vi "Condition _string_For_Month.vi"(0 "Select Line 2":string(combo)="ST 1", 1 "connection reference":T1, 2 "Shift":string(combo)="ALL", 3 "BREAKDOWN_STK_HOLD_ID":i32=1, 4 "Found Date":string[](array[string]), 5 "year":string(combo)="ST 1", 6 "month":string, 7 "error in (no error)":errorcluster) -> (12 "Duration count":string[][](array[string]), 13 "error out":errorcluster, 15 "connection reference 2":T1, 18 "BD Count":string[][](array[string]))   [LabVIEW 2017]
uses:
  <vilib>/addons/database/Connection.llb/Conn ObjectReference.ctl
  <vilib>/addons/database/NI_Database_API.lvlib
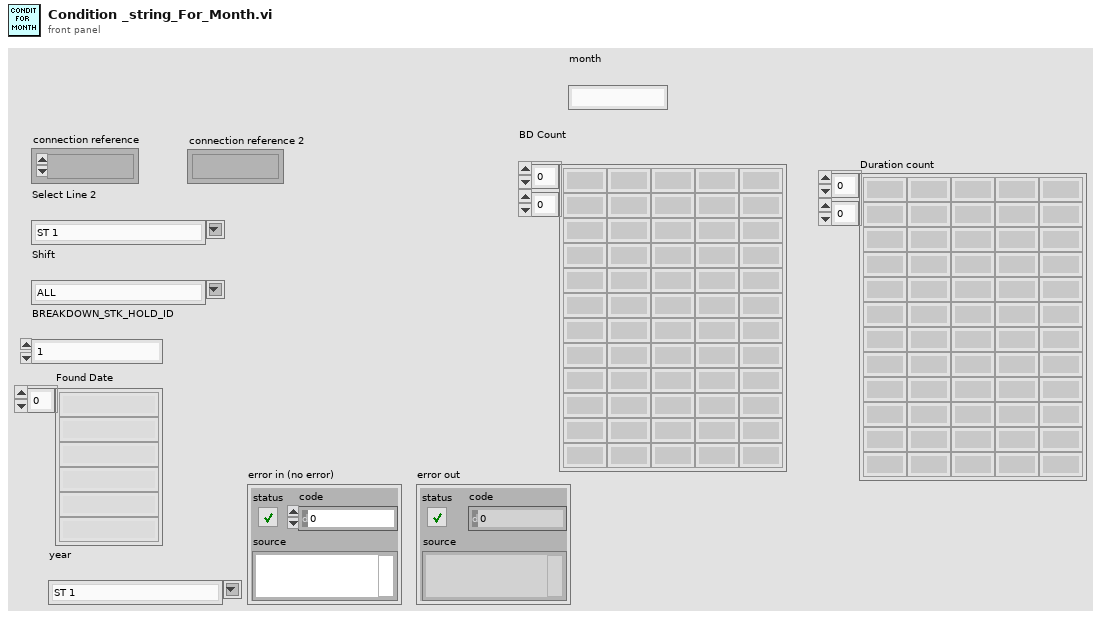
[diagram p1: front panel]
types:
  T1 = typedef "NI_Database_API.lvlib/Conn ObjectReference.ctl" = refnum<k1>
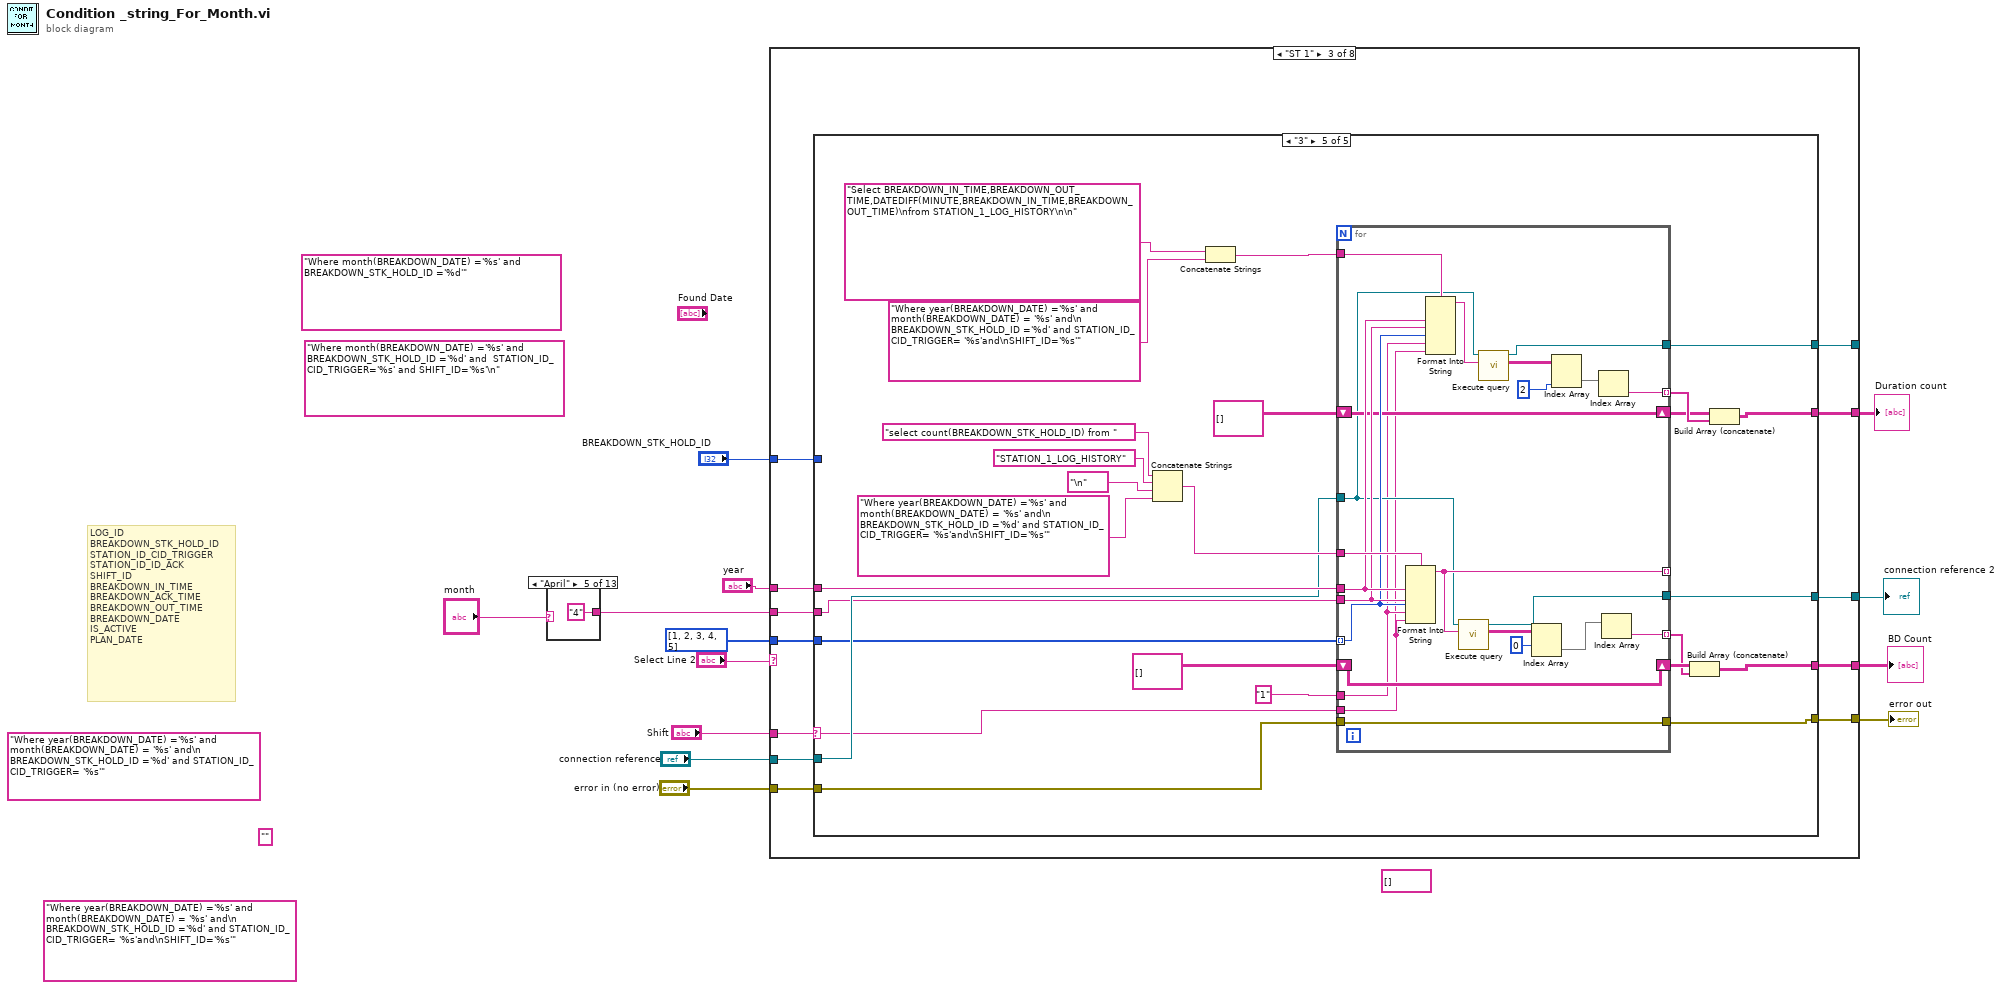
[diagram p0: block diagram]
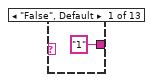
[diagram p2: hidden frame]
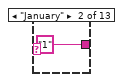
[diagram p3: hidden frame]
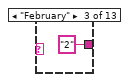
[diagram p4: hidden frame]
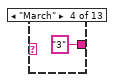
[diagram p5: hidden frame]
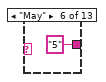
[diagram p6: hidden frame]
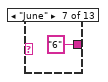
[diagram p7: hidden frame]
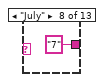
[diagram p8: hidden frame]
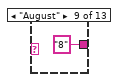
[diagram p9: hidden frame]
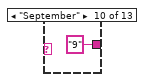
[diagram p10: hidden frame]
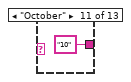
[diagram p11: hidden frame]
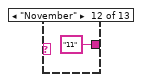
[diagram p12: hidden frame]
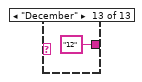
[diagram p13: hidden frame]
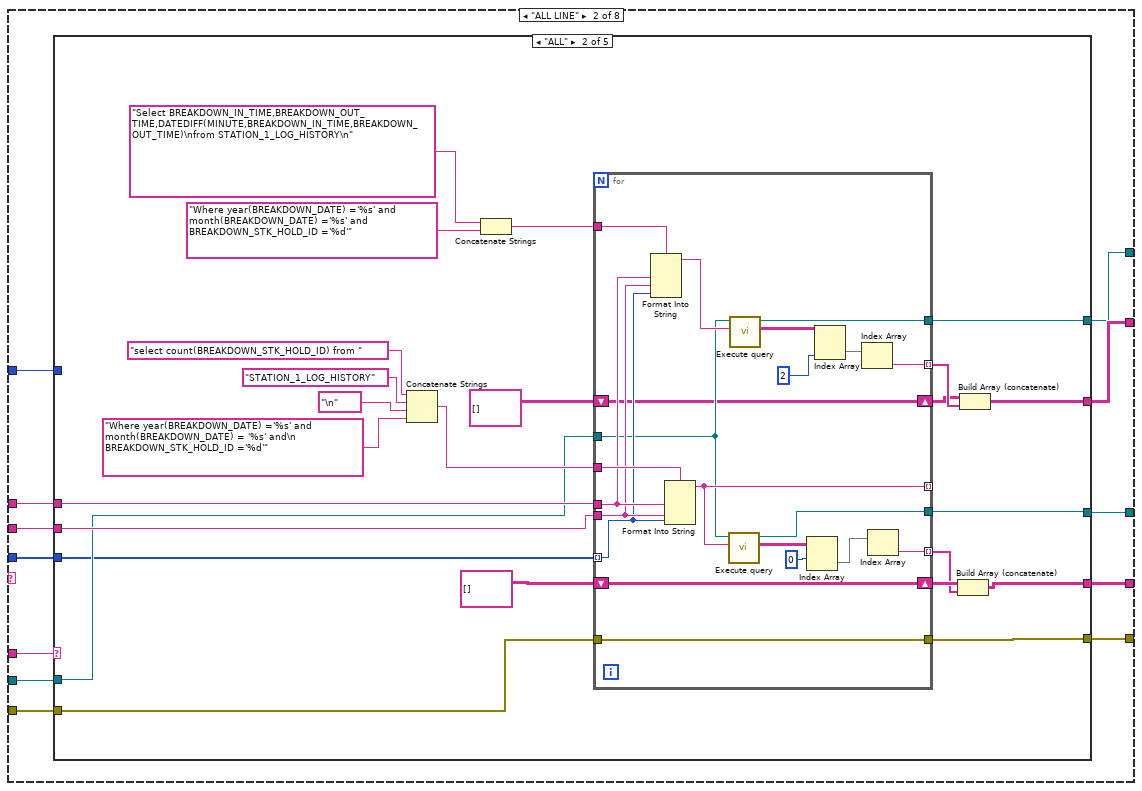
[diagram p15: hidden frame]
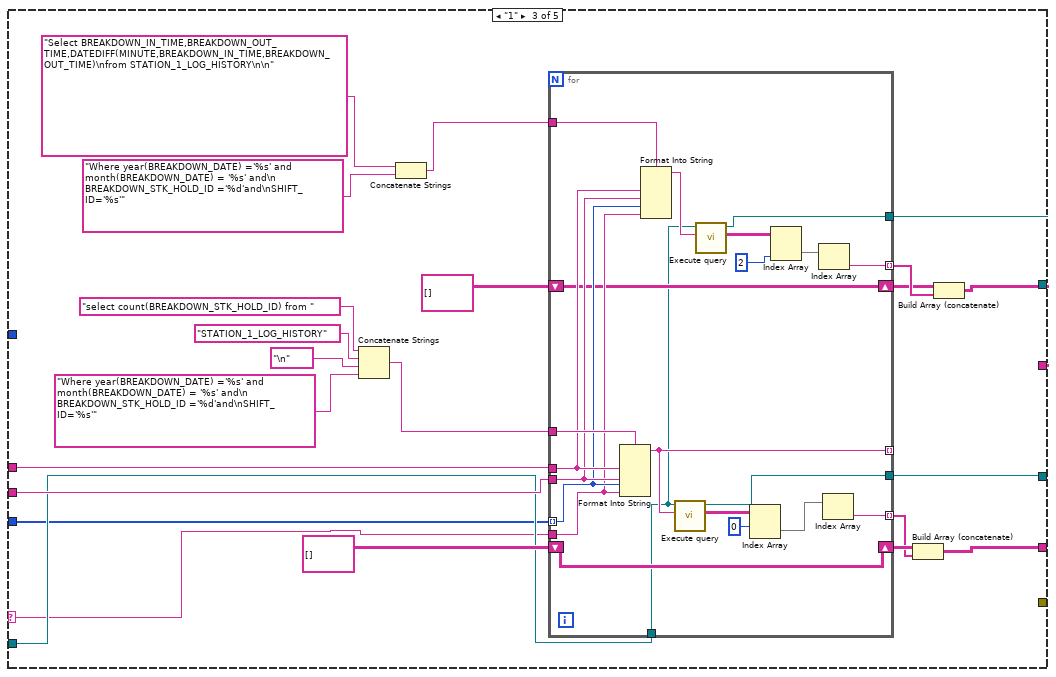
[diagram p17: hidden frame]
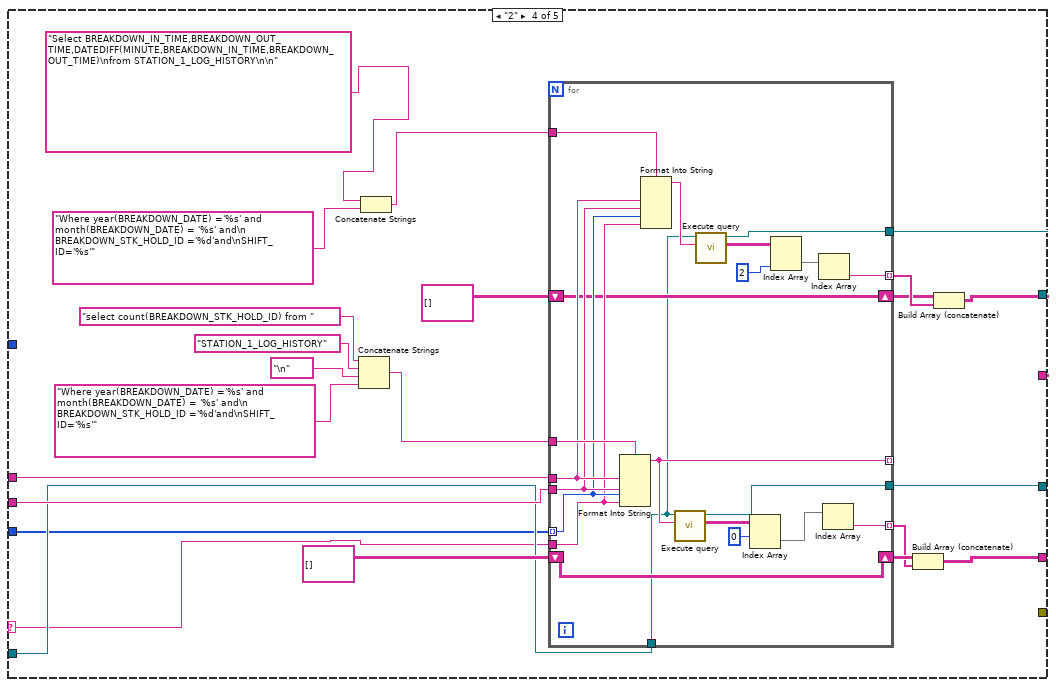
[diagram p18: hidden frame]
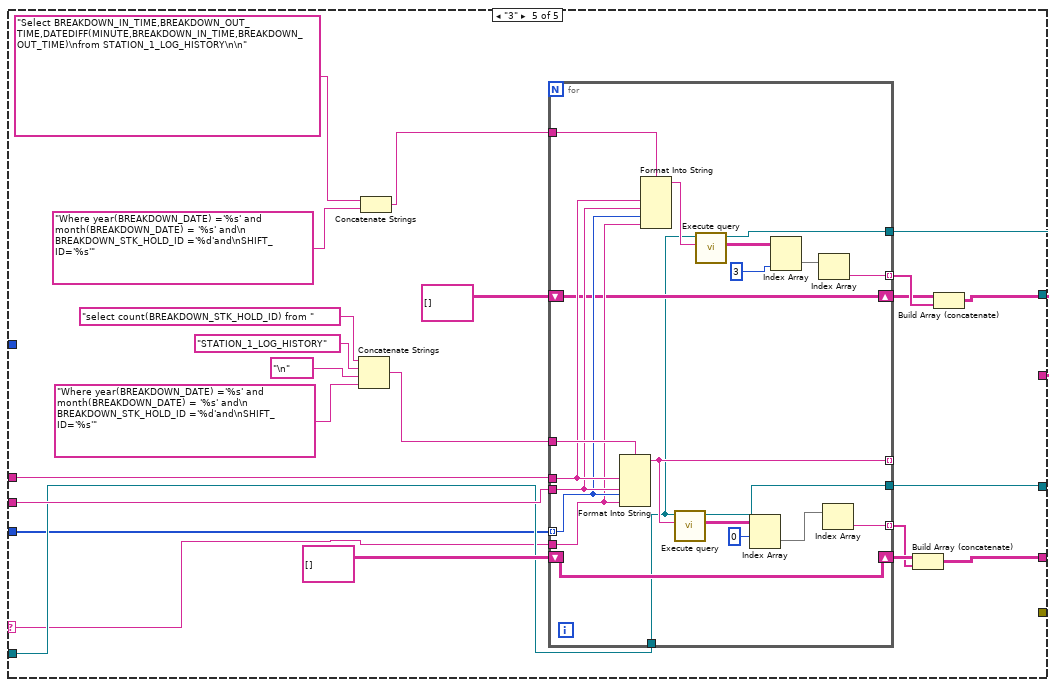
[diagram p19: hidden frame]
diagram:
  (unwired) "Where month(BREAKDOWN_DATE) ='%s' and  BREAKDOWN_STK_HOLD_ID ='%d'" ("condition")
  (unwired) "Where month(BREAKDOWN_DATE) ='%s' and  BREAKDOWN_STK_HOLD_ID ='%d' and  STATION_ID_CID_TRIGGER='%s' and SHIFT_ID='%s'\n" ("condition")
  (unwired) ""
  (unwired) "Where year(BREAKDOWN_DATE) ='%s' and month(BREAKDOWN_DATE) = '%s' and\n BREAKDOWN_STK_HOLD_ID ='%d' and STATION_ID_CID_TRIGGER= '%s'and\nSHIFT_ID='%s'" ("condition")
  (unwired) "Where year(BREAKDOWN_DATE) ='%s' and month(BREAKDOWN_DATE) = '%s' and\n BREAKDOWN_STK_HOLD_ID ='%d' and STATION_ID_CID_TRIGGER= '%s'" ("condition")
  (unwired) string[] [] ("Output Array")
  # "LOG_ID\nBREAKDOWN_STK_HOLD_ID\nSTATION_ID_CID_TRIGGER\nSTATION_ID_ID_ACK\nSHIFT_ID\nBREAKDOWN_IN_TIME\nBREAKDOWN_ACK_TIME\nBREAKDOWN_OUT_TIME\nBREAKDOWN_DATE\nIS_ACTIVE\nPLAN_DATE"
  n1 = case shown="\"April\"" "month" {
    tunnel: ["1" "1" "2" "3" "4" "5" "6" "7" "8" "9" "10" "11" "12"] -> w1
    frame "False", Default {
    }
    frame "January" {
    }
    frame "February" {
    }
    frame "March" {
    }
    frame "April" {
    }
    frame "May" {
    }
    frame "June" {
    }
    frame "July" {
    }
    frame "August" {
    }
    frame "September" {
    }
    frame "October" {
    }
    frame "November" {
    }
    frame "December" {
    }
  }
  n2 = case shown="\"ST 1\"" "Select Line 2" {
    tunnel: "Shift" -> [_ w38 w229 w437 w717 w997 w1277 w1560]
    tunnel: "BREAKDOWN_STK_HOLD_ID" -> [_ w37 w228 w436 w716 w996 w1276 w1559]
    tunnel: "year" -> [_ w36 w227 w435 w715 w995 w1275 w1558]
    tunnel: w1 -> [_ w35 w226 w434 w714 w994 w1274 w1557]
    tunnel: [_ w34 w225 w433 w713 w993 w1273 w1556] -> w9
    tunnel: "connection reference" -> [_ w33 w224 w432 w712 w992 w1272 w1555]
    tunnel: [_ w32 w223 w431 w711 w991 w1271 w1554] -> w7
    tunnel: i32[] [1, 2, 3, 4, 5] -> [_ w31 w222 w430 w710 w990 w1270 w1553]
    tunnel: [_ w30 w221 w429 w709 w989 w1269 w1552] -> w5
    tunnel: [_ w29 w220 w428 w708 w988 w1268 w1551] -> _
    tunnel: "error in (no error)" -> [_ w28 w219 w427 w707 w987 w1267 w1550]
    tunnel: [_ w27 w218 w426 w706 w986 w1266 w1549] -> w3
    frame "False", Default {
    }
    frame "ALL LINE" {
      n3 = case shown="\"ALL\"" w38 {
        selector: w38 -> [_ _ w96 w140 w184]
        tunnel: w37 -> [_ _ _ _ _]
        tunnel: w36 -> [_ w59 w103 w147 w191]
        tunnel: w35 -> [_ w56 w100 w144 w188]
        tunnel: [_ w60 w104 w148 w192] -> w34
        tunnel: w33 -> [w40 w55 w99 w143 w187]
        tunnel: [w40 w54 w98 w142 w186] -> w32
        tunnel: w31 -> [_ w53 w97 w141 w185]
        tunnel: [_ w49 w93 w136 w180] -> w30
        tunnel: [_ w48 w92 w135 w179] -> w29
        tunnel: w28 -> [w39 w46 _ _ _]
        tunnel: [w39 w45 _ _ _] -> w27
        frame "False", Default {
        }
        frame "ALL" {
          n4 = Concatenate Strings("select count(BREAKDOWN_STK_HOLD_ID) from " ("string"), "STATION_1_LOG_HISTORY" ("table"), "\n" ("string"), "Where year(BREAKDOWN_DATE) ='%s' and month(BREAKDOWN_DATE) = '%s' and\n BREAKDOWN_STK_HOLD_ID ='%d'" ("condition")) -> (w58:string)
          n5 = Concatenate Strings("Select BREAKDOWN_IN_TIME,BREAKDOWN_OUT_TIME,DATEDIFF(MINUTE,BREAKDOWN_IN_TIME,BREAKDOWN_OUT_TIME)\nfrom STATION_1_LOG_HISTORY\n" ("string"), "Where year(BREAKDOWN_DATE) ='%s' and month(BREAKDOWN_DATE) ='%s' and BREAKDOWN_STK_HOLD_ID ='%d'" ("condition")) -> (w51:string)
          n6 = for {
            tunnel: w58 -> [w85]
            tunnel: w59 -> [w75]
            tunnel: w56 -> [w74]
            tunnel: [w84] -> _ mode=indexing
            tunnel: w55 -> [w72]
            tunnel: [w82] -> w54
            tunnel: w53 -> [w73] mode=indexing
            shift-right: [w83] -> w44
            shift-left: string[][] [] ("Output Array") -> [w83]
            tunnel: [w78] -> w43 mode=indexing
            tunnel: w51 -> [w76]
            tunnel: [w69] -> w48
            tunnel: [w68] -> w42 mode=indexing
            shift-right: [w67] -> w41
            shift-left: string[][] [] ("Output Array") -> [w67]
            tunnel: [w65] -> w45
            tunnel: w46 -> [w65]
            n7 = Format Into String(format string=w76, w75, w74, w73) -> (resulting string=w77:string)  [unwired: 2 in, 1 out]
            n8 = Format Into String(format string=w85, w75, w74, w73) -> (resulting string=w84:string)  [unwired: 2 in, 1 out]
            n9 = call "Execute query.vi"("String"=w84, "connection reference"=w72) -> ("Table"=w81:string[][], "connection reference 2"=w82:T1)  [unwired: 6 in, 2 out]
            n10 = call "Execute query.vi"("String"=w77, "connection reference"=w72) -> ("Table"=w71:string[][], "connection reference 2"=w69:T1)  [unwired: 6 in, 2 out]
            n11 = Index Array(array=w81, index (row)=0 ("disabled index (col)")) -> (element=w79:string[])  [unwired: 1 in]
            n12 = Index Array(array=w71, index (col)=2 ("disabled index (col)")) -> (element=w70:string[])  [unwired: 1 in]
            n13 = Index Array(array=w70) -> (element=w68:string)  [unwired: 1 in]
            n14 = Index Array(array=w79) -> (element=w78:string)  [unwired: 1 in]
          }
          n15 = Build Array (concatenate)(w44, w43) -> (w60:string[][])
          n16 = Build Array (concatenate)(w41, w42) -> (w49:string[][])
        }
        frame "1" {
          n17 = Concatenate Strings("select count(BREAKDOWN_STK_HOLD_ID) from " ("string"), "STATION_1_LOG_HISTORY" ("table"), "\n" ("string"), "Where year(BREAKDOWN_DATE) ='%s' and month(BREAKDOWN_DATE) = '%s' and\n BREAKDOWN_STK_HOLD_ID ='%d'and\nSHIFT_ID='%s'" ("condition")) -> (w102:string)
          n18 = Concatenate Strings("Select BREAKDOWN_IN_TIME,BREAKDOWN_OUT_TIME,DATEDIFF(MINUTE,BREAKDOWN_IN_TIME,BREAKDOWN_OUT_TIME)\nfrom STATION_1_LOG_HISTORY\n\n" ("string"), "Where year(BREAKDOWN_DATE) ='%s' and month(BREAKDOWN_DATE) = '%s' and\n BREAKDOWN_STK_HOLD_ID ='%d'and\nSHIFT_ID='%s'" ("condition")) -> (w91:string)
          n19 = for {
            tunnel: w102 -> [w129]
            tunnel: w103 -> [w117]
            tunnel: w100 -> [w116]
            tunnel: [w128] -> _ mode=indexing
            tunnel: w99 -> [w111]
            tunnel: [w126] -> w98
            tunnel: w97 -> [w115] mode=indexing
            shift-right: [w127] -> w89
            shift-left: string[][] [] ("Output Array") -> [w127]
            tunnel: [w123] -> w88 mode=indexing
            tunnel: w96 -> [w114]
            tunnel: w91 -> [w118]
            tunnel: [w113] -> w87 mode=indexing
            shift-right: [w112] -> w86
            shift-left: string[][] [] ("Output Array") -> [w112]
            tunnel: [w110] -> w92
            n20 = Format Into String(format string=w129, w117, w116, w115, w114) -> (resulting string=w128:string)  [unwired: 2 in, 1 out]
            n21 = Format Into String(format string=w118, w117, w116, w115, w114) -> (resulting string=w121:string)  [unwired: 2 in, 1 out]
            n22 = call "Execute query.vi"("String"=w128, "connection reference"=w111) -> ("Table"=w122:string[][], "connection reference 2"=w126:T1)  [unwired: 6 in, 2 out]
            n23 = call "Execute query.vi"("String"=w121, "connection reference"=w111) -> ("Table"=w119:string[][], "connection reference 2"=w110:T1)  [unwired: 6 in, 2 out]
            n24 = Index Array(array=w122, index (row)=0 ("disabled index (col)")) -> (element=w124:string[])  [unwired: 1 in]
            n25 = Index Array(array=w119, index (col)=2 ("disabled index (col)")) -> (element=w120:string[])  [unwired: 1 in]
            n26 = Index Array(array=w120) -> (element=w113:string)  [unwired: 1 in]
            n27 = Index Array(array=w124) -> (element=w123:string)  [unwired: 1 in]
          }
          n28 = Build Array (concatenate)(w89, w88) -> (w104:string[][])
          n29 = Build Array (concatenate)(w86, w87) -> (w93:string[][])
        }
        frame "2" {
          n30 = Concatenate Strings("select count(BREAKDOWN_STK_HOLD_ID) from " ("string"), "STATION_1_LOG_HISTORY" ("table"), "\n" ("string"), "Where year(BREAKDOWN_DATE) ='%s' and month(BREAKDOWN_DATE) = '%s' and\n BREAKDOWN_STK_HOLD_ID ='%d'and\nSHIFT_ID='%s'" ("condition")) -> (w146:string)
          n31 = Concatenate Strings("Select BREAKDOWN_IN_TIME,BREAKDOWN_OUT_TIME,DATEDIFF(MINUTE,BREAKDOWN_IN_TIME,BREAKDOWN_OUT_TIME)\nfrom STATION_1_LOG_HISTORY\n\n" ("string"), "Where year(BREAKDOWN_DATE) ='%s' and month(BREAKDOWN_DATE) = '%s' and\n BREAKDOWN_STK_HOLD_ID ='%d'and\nSHIFT_ID='%s'" ("condition")) -> (w138:string)
          n32 = for {
            tunnel: w146 -> [w173]
            tunnel: w147 -> [w161]
            tunnel: w144 -> [w160]
            tunnel: [w172] -> _ mode=indexing
            tunnel: w143 -> [w155]
            tunnel: [w170] -> w142
            tunnel: w141 -> [w159] mode=indexing
            shift-right: [w171] -> w133
            shift-left: string[][] [] ("Output Array") -> [w171]
            tunnel: [w167] -> w132 mode=indexing
            tunnel: w140 -> [w158]
            tunnel: w138 -> [w162]
            tunnel: [w157] -> w131 mode=indexing
            shift-right: [w156] -> w130
            shift-left: string[][] [] ("Output Array") -> [w156]
            tunnel: [w154] -> w135
            n33 = Format Into String(format string=w173, w161, w160, w159, w158) -> (resulting string=w172:string)  [unwired: 2 in, 1 out]
            n34 = Format Into String(format string=w162, w161, w160, w159, w158) -> (resulting string=w165:string)  [unwired: 2 in, 1 out]
            n35 = call "Execute query.vi"("String"=w172, "connection reference"=w155) -> ("Table"=w166:string[][], "connection reference 2"=w170:T1)  [unwired: 6 in, 2 out]
            n36 = call "Execute query.vi"("String"=w165, "connection reference"=w155) -> ("Table"=w163:string[][], "connection reference 2"=w154:T1)  [unwired: 6 in, 2 out]
            n37 = Index Array(array=w166, index (row)=0 ("disabled index (col)")) -> (element=w168:string[])  [unwired: 1 in]
            n38 = Index Array(array=w163, index (col)=2 ("disabled index (col)")) -> (element=w164:string[])  [unwired: 1 in]
            n39 = Index Array(array=w164) -> (element=w157:string)  [unwired: 1 in]
            n40 = Index Array(array=w168) -> (element=w167:string)  [unwired: 1 in]
          }
          n41 = Build Array (concatenate)(w133, w132) -> (w148:string[][])
          n42 = Build Array (concatenate)(w130, w131) -> (w136:string[][])
        }
        frame "3" {
          n43 = Concatenate Strings("select count(BREAKDOWN_STK_HOLD_ID) from " ("string"), "STATION_1_LOG_HISTORY" ("table"), "\n" ("string"), "Where year(BREAKDOWN_DATE) ='%s' and month(BREAKDOWN_DATE) = '%s' and\n BREAKDOWN_STK_HOLD_ID ='%d'and\nSHIFT_ID='%s'" ("condition")) -> (w190:string)
          n44 = Concatenate Strings("Select BREAKDOWN_IN_TIME,BREAKDOWN_OUT_TIME,DATEDIFF(MINUTE,BREAKDOWN_IN_TIME,BREAKDOWN_OUT_TIME)\nfrom STATION_1_LOG_HISTORY\n\n" ("string"), "Where year(BREAKDOWN_DATE) ='%s' and month(BREAKDOWN_DATE) = '%s' and\n BREAKDOWN_STK_HOLD_ID ='%d'and\nSHIFT_ID='%s'" ("condition")) -> (w182:string)
          n45 = for {
            tunnel: w190 -> [w217]
            tunnel: w191 -> [w206]
            tunnel: w188 -> [w205]
            tunnel: [w216] -> _ mode=indexing
            tunnel: w187 -> [w198]
            tunnel: [w214] -> w186
            tunnel: w185 -> [w204] mode=indexing
            shift-right: [w215] -> w177
            shift-left: string[][] [] ("Output Array") -> [w215]
            tunnel: [w212] -> w176 mode=indexing
            tunnel: w184 -> [w203]
            tunnel: w182 -> [w207]
            tunnel: [w202] -> w175 mode=indexing
            shift-right: [w201] -> w174
            shift-left: string[][] [] ("Output Array") -> [w201]
            tunnel: [w199] -> w179
            n46 = Format Into String(format string=w217, w206, w205, w204, w203) -> (resulting string=w216:string)  [unwired: 2 in, 1 out]
            n47 = Format Into String(format string=w207, w206, w205, w204, w203) -> (resulting string=w210:string)  [unwired: 2 in, 1 out]
            n48 = call "Execute query.vi"("String"=w216, "connection reference"=w198) -> ("Table"=w211:string[][], "connection reference 2"=w214:T1)  [unwired: 6 in, 2 out]
            n49 = call "Execute query.vi"("String"=w210, "connection reference"=w198) -> ("Table"=w208:string[][], "connection reference 2"=w199:T1)  [unwired: 6 in, 2 out]
            n50 = Index Array(array=w211, index (row)=0 ("disabled index (col)")) -> (element=w200:string[])  [unwired: 1 in]
            n51 = Index Array(array=w208, index (col)=3 ("disabled index (col)")) -> (element=w209:string[])  [unwired: 1 in]
            n52 = Index Array(array=w209) -> (element=w202:string)  [unwired: 1 in]
            n53 = Index Array(array=w200) -> (element=w212:string)  [unwired: 1 in]
          }
          n54 = Build Array (concatenate)(w177, w176) -> (w192:string[][])
          n55 = Build Array (concatenate)(w174, w175) -> (w180:string[][])
        }
      }
    }
    frame "ST 1" {
      n56 = case shown="\"3\"" w229 {
        selector: w229 -> [_ _ w287 w336 w385]
        tunnel: w228 -> [_ _ _ _ _]
        tunnel: w227 -> [_ w252 w300 w349 w398]
        tunnel: w226 -> [_ w249 w279 w328 w377]
        tunnel: [_ w253 w301 w350 w399] -> w225
        tunnel: w224 -> [w231 w248 w297 w346 w395]
        tunnel: [w231 w247 w296 w345 w394] -> w223
        tunnel: w222 -> [_ w246 w295 w344 w393]
        tunnel: [_ w243 w293 w342 w391] -> w221
        tunnel: [_ w242 w292 w341 w390] -> w220
        tunnel: w219 -> [w230 w240 w284 w333 w382]
        tunnel: [w230 w239 w285 w334 w383] -> w218
        frame "False", Default {
        }
        frame "ALL" {
          n57 = Concatenate Strings("select count(BREAKDOWN_STK_HOLD_ID) from " ("string"), "STATION_1_LOG_HISTORY" ("table"), "\n" ("string"), "Where year(BREAKDOWN_DATE) ='%s' and month(BREAKDOWN_DATE) = '%s' and\n BREAKDOWN_STK_HOLD_ID ='%d' and STATION_ID_CID_TRIGGER= '%s'" ("condition")) -> (w251:string)
          n58 = Concatenate Strings("Select BREAKDOWN_IN_TIME,BREAKDOWN_OUT_TIME,DATEDIFF(MINUTE,BREAKDOWN_IN_TIME,BREAKDOWN_OUT_TIME)\nfrom STATION_1_LOG_HISTORY\n" ("string"), "Where year(BREAKDOWN_DATE) ='%s' and month(BREAKDOWN_DATE) = '%s' and\n BREAKDOWN_STK_HOLD_ID ='%d' and STATION_ID_CID_TRIGGER= '%s'" ("condition")) -> (w245:string)
          n59 = for {
            tunnel: w251 -> [w278]
            tunnel: w252 -> [w268]
            tunnel: w249 -> [w267]
            tunnel: [w277] -> _ mode=indexing
            tunnel: w248 -> [w265]
            tunnel: [w275] -> w247
            tunnel: w246 -> [w266] mode=indexing
            shift-right: [w276] -> w235
            shift-left: string[][] [] ("Output Array") -> [w276]
            tunnel: [w271] -> w234 mode=indexing
            tunnel: w245 -> [w269]
            tunnel: [w262] -> w242
            tunnel: [w261] -> w233 mode=indexing
            shift-right: [w260] -> w232
            shift-left: string[][] [] ("Output Array") -> [w260]
            tunnel: [w258] -> w239
            tunnel: w240 -> [w258]
            tunnel: "1" -> [w257]
            n60 = Format Into String(format string=w269, w268, w267, w266, w257) -> (resulting string=w270:string)  [unwired: 2 in, 1 out]
            n61 = Format Into String(format string=w278, w268, w267, w266, w257) -> (resulting string=w277:string)  [unwired: 2 in, 1 out]
            n62 = call "Execute query.vi"("String"=w277, "connection reference"=w265) -> ("Table"=w274:string[][], "connection reference 2"=w275:T1)  [unwired: 6 in, 2 out]
            n63 = call "Execute query.vi"("String"=w270, "connection reference"=w265) -> ("Table"=w264:string[][], "connection reference 2"=w262:T1)  [unwired: 6 in, 2 out]
            n64 = Index Array(array=w274, index (row)=0 ("disabled index (col)")) -> (element=w272:string[])  [unwired: 1 in]
            n65 = Index Array(array=w264, index (col)=2 ("disabled index (col)")) -> (element=w263:string[])  [unwired: 1 in]
            n66 = Index Array(array=w263) -> (element=w261:string)  [unwired: 1 in]
            n67 = Index Array(array=w272) -> (element=w271:string)  [unwired: 1 in]
          }
          n68 = Build Array (concatenate)(w235, w234) -> (w253:string[][])
          n69 = Build Array (concatenate)(w232, w233) -> (w243:string[][])
        }
        frame "1" {
          n70 = Concatenate Strings("select count(BREAKDOWN_STK_HOLD_ID) from " ("string"), "STATION_1_LOG_HISTORY" ("table"), "\n" ("string"), "Where year(BREAKDOWN_DATE) ='%s' and month(BREAKDOWN_DATE) = '%s' and\n BREAKDOWN_STK_HOLD_ID ='%d' and STATION_ID_CID_TRIGGER= '%s'and\nSHIFT_ID='%s'" ("condition")) -> (w299:string)
          n71 = Concatenate Strings("Select BREAKDOWN_IN_TIME,BREAKDOWN_OUT_TIME,DATEDIFF(MINUTE,BREAKDOWN_IN_TIME,BREAKDOWN_OUT_TIME)\nfrom STATION_1_LOG_HISTORY\n\n" ("string"), "Where year(BREAKDOWN_DATE) ='%s' and month(BREAKDOWN_DATE) = '%s' and\n BREAKDOWN_STK_HOLD_ID ='%d' and STATION_ID_CID_TRIGGER= '%s'and\nSHIFT_ID='%s'" ("condition")) -> (w291:string)
          n72 = for {
            tunnel: w299 -> [w327]
            tunnel: w300 -> [w315]
            tunnel: w279 -> [w314]
            tunnel: [w326] -> _ mode=indexing
            tunnel: w297 -> [w310]
            tunnel: [w324] -> w296
            tunnel: w295 -> [w313] mode=indexing
            shift-right: [w325] -> w283
            shift-left: string[][] [] ("Output Array") -> [w325]
            tunnel: [w321] -> w282 mode=indexing
            tunnel: w291 -> [w316]
            tunnel: [w312] -> w281 mode=indexing
            shift-right: [w311] -> w280
            shift-left: string[][] [] ("Output Array") -> [w311]
            tunnel: [w309] -> w292
            tunnel: "1" -> [w307]
            tunnel: w287 -> [w306]
            tunnel: [w305] -> w285
            tunnel: w284 -> [w305]
            n73 = Format Into String(format string=w327, w315, w314, w313, w307, w306) -> (resulting string=w326:string)  [unwired: 2 in, 1 out]
            n74 = Format Into String(format string=w316, w315, w314, w313, w307, w306) -> (resulting string=w319:string)  [unwired: 2 in, 1 out]
            n75 = call "Execute query.vi"("String"=w326, "connection reference"=w310) -> ("Table"=w320:string[][], "connection reference 2"=w324:T1)  [unwired: 6 in, 2 out]
            n76 = call "Execute query.vi"("String"=w319, "connection reference"=w310) -> ("Table"=w317:string[][], "connection reference 2"=w309:T1)  [unwired: 6 in, 2 out]
            n77 = Index Array(array=w320, index (row)=0 ("disabled index (col)")) -> (element=w322:string[])  [unwired: 1 in]
            n78 = Index Array(array=w317, index (col)=2 ("disabled index (col)")) -> (element=w318:string[])  [unwired: 1 in]
            n79 = Index Array(array=w318) -> (element=w312:string)  [unwired: 1 in]
            n80 = Index Array(array=w322) -> (element=w321:string)  [unwired: 1 in]
          }
          n81 = Build Array (concatenate)(w283, w282) -> (w301:string[][])
          n82 = Build Array (concatenate)(w280, w281) -> (w293:string[][])
        }
        frame "2" {
          n83 = Concatenate Strings("select count(BREAKDOWN_STK_HOLD_ID) from " ("string"), "STATION_1_LOG_HISTORY" ("table"), "\n" ("string"), "Where year(BREAKDOWN_DATE) ='%s' and month(BREAKDOWN_DATE) = '%s' and\n BREAKDOWN_STK_HOLD_ID ='%d' and STATION_ID_CID_TRIGGER= '%s'and\nSHIFT_ID='%s'" ("condition")) -> (w348:string)
          n84 = Concatenate Strings("Select BREAKDOWN_IN_TIME,BREAKDOWN_OUT_TIME,DATEDIFF(MINUTE,BREAKDOWN_IN_TIME,BREAKDOWN_OUT_TIME)\nfrom STATION_1_LOG_HISTORY\n\n" ("string"), "Where year(BREAKDOWN_DATE) ='%s' and month(BREAKDOWN_DATE) = '%s' and\n BREAKDOWN_STK_HOLD_ID ='%d' and STATION_ID_CID_TRIGGER= '%s'and\nSHIFT_ID='%s'" ("condition")) -> (w340:string)
          n85 = for {
            tunnel: w348 -> [w376]
            tunnel: w349 -> [w364]
            tunnel: w328 -> [w363]
            tunnel: [w375] -> _ mode=indexing
            tunnel: w346 -> [w359]
            tunnel: [w373] -> w345
            tunnel: w344 -> [w362] mode=indexing
            shift-right: [w374] -> w332
            shift-left: string[][] [] ("Output Array") -> [w374]
            tunnel: [w370] -> w331 mode=indexing
            tunnel: w340 -> [w365]
            tunnel: [w361] -> w330 mode=indexing
            shift-right: [w360] -> w329
            shift-left: string[][] [] ("Output Array") -> [w360]
            tunnel: [w358] -> w341
            tunnel: "1" -> [w356]
            tunnel: w336 -> [w355]
            tunnel: [w354] -> w334
            tunnel: w333 -> [w354]
            n86 = Format Into String(format string=w376, w364, w363, w362, w356, w355) -> (resulting string=w375:string)  [unwired: 2 in, 1 out]
            n87 = Format Into String(format string=w365, w364, w363, w362, w356, w355) -> (resulting string=w368:string)  [unwired: 2 in, 1 out]
            n88 = call "Execute query.vi"("String"=w375, "connection reference"=w359) -> ("Table"=w369:string[][], "connection reference 2"=w373:T1)  [unwired: 6 in, 2 out]
            n89 = call "Execute query.vi"("String"=w368, "connection reference"=w359) -> ("Table"=w366:string[][], "connection reference 2"=w358:T1)  [unwired: 6 in, 2 out]
            n90 = Index Array(array=w369, index (row)=0 ("disabled index (col)")) -> (element=w371:string[])  [unwired: 1 in]
            n91 = Index Array(array=w366, index (col)=2 ("disabled index (col)")) -> (element=w367:string[])  [unwired: 1 in]
            n92 = Index Array(array=w367) -> (element=w361:string)  [unwired: 1 in]
            n93 = Index Array(array=w371) -> (element=w370:string)  [unwired: 1 in]
          }
          n94 = Build Array (concatenate)(w332, w331) -> (w350:string[][])
          n95 = Build Array (concatenate)(w329, w330) -> (w342:string[][])
        }
        frame "3" {
          n96 = Concatenate Strings("select count(BREAKDOWN_STK_HOLD_ID) from " ("string"), "STATION_1_LOG_HISTORY" ("table"), "\n" ("string"), "Where year(BREAKDOWN_DATE) ='%s' and month(BREAKDOWN_DATE) = '%s' and\n BREAKDOWN_STK_HOLD_ID ='%d' and STATION_ID_CID_TRIGGER= '%s'and\nSHIFT_ID='%s'" ("condition")) -> (w397:string)
          n97 = Concatenate Strings("Select BREAKDOWN_IN_TIME,BREAKDOWN_OUT_TIME,DATEDIFF(MINUTE,BREAKDOWN_IN_TIME,BREAKDOWN_OUT_TIME)\nfrom STATION_1_LOG_HISTORY\n\n" ("string"), "Where year(BREAKDOWN_DATE) ='%s' and month(BREAKDOWN_DATE) = '%s' and\n BREAKDOWN_STK_HOLD_ID ='%d' and STATION_ID_CID_TRIGGER= '%s'and\nSHIFT_ID='%s'" ("condition")) -> (w389:string)
          n98 = for {
            tunnel: w397 -> [w425]
            tunnel: w398 -> [w413]
            tunnel: w377 -> [w412]
            tunnel: [w424] -> _ mode=indexing
            tunnel: w395 -> [w408]
            tunnel: [w422] -> w394
            tunnel: w393 -> [w411] mode=indexing
            shift-right: [w423] -> w381
            shift-left: string[][] [] ("Output Array") -> [w423]
            tunnel: [w419] -> w380 mode=indexing
            tunnel: w389 -> [w414]
            tunnel: [w410] -> w379 mode=indexing
            shift-right: [w409] -> w378
            shift-left: string[][] [] ("Output Array") -> [w409]
            tunnel: [w407] -> w390
            tunnel: "1" -> [w405]
            tunnel: w385 -> [w404]
            tunnel: [w403] -> w383
            tunnel: w382 -> [w403]
            n99 = Format Into String(format string=w425, w413, w412, w411, w405, w404) -> (resulting string=w424:string)  [unwired: 2 in, 1 out]
            n100 = Format Into String(format string=w414, w413, w412, w411, w405, w404) -> (resulting string=w417:string)  [unwired: 2 in, 1 out]
            n101 = call "Execute query.vi"("String"=w424, "connection reference"=w408) -> ("Table"=w418:string[][], "connection reference 2"=w422:T1)  [unwired: 6 in, 2 out]
            n102 = call "Execute query.vi"("String"=w417, "connection reference"=w408) -> ("Table"=w415:string[][], "connection reference 2"=w407:T1)  [unwired: 6 in, 2 out]
            n103 = Index Array(array=w418, index (row)=0 ("disabled index (col)")) -> (element=w420:string[])  [unwired: 1 in]
            n104 = Index Array(array=w415, index (col)=2 ("disabled index (col)")) -> (element=w416:string[])  [unwired: 1 in]
            n105 = Index Array(array=w416) -> (element=w410:string)  [unwired: 1 in]
            n106 = Index Array(array=w420) -> (element=w419:string)  [unwired: 1 in]
          }
          n107 = Build Array (concatenate)(w381, w380) -> (w399:string[][])
          n108 = Build Array (concatenate)(w378, w379) -> (w391:string[][])
        }
      }
    }
    frame "ST 2" {
      n109 = disable-structure shown="Disabled" {
        disable-tunnel: w437 -> [w449 _]
        disable-tunnel: w436 -> [w448 _]
        disable-tunnel: w435 -> [w447 _]
        disable-tunnel: w434 -> [w446 _]
        disable-tunnel: [w445 _] -> w433
        disable-tunnel: w432 -> [w444 _]
        disable-tunnel: [w443 _] -> w431
        disable-tunnel: w430 -> [w442 _]
        disable-tunnel: [w441 _] -> w429
        disable-tunnel: [w440 _] -> w428
        disable-tunnel: w427 -> [w439 _]
        disable-tunnel: [w438 _] -> w426
        frame Disabled {
          n110 = case shown="\"ALL\"" w449 {
            selector: w449 -> [_ _ w517 w581 w645]
            tunnel: w448 -> [_ _ _ _ _]
            tunnel: w447 -> [_ w468 w531 w595 w659]
            tunnel: w446 -> [_ w465 _ _ _]
            tunnel: [_ w469 w532 w596 w660] -> w445
            tunnel: w444 -> [w451 w464 w527 w591 w655]
            tunnel: [w451 w463 w526 w590 w654] -> w443
            tunnel: w442 -> [_ w462 w525 w589 w653]
            tunnel: [_ w459 w523 w587 w651] -> w441
            tunnel: [_ w458 w522 w586 w650] -> w440
            tunnel: w439 -> [w450 w456 w514 w578 w642]
            tunnel: [w450 w455 w515 w579 w643] -> w438
            frame "False", Default {
            }
            frame "ALL" {
              n111 = Concatenate Strings("select count(BREAKDOWN_STK_HOLD_ID) from " ("string"), "STATION_1_LOG_HISTORY" ("table"), "\n" ("string"), "Where year(BREAKDOWN_DATE) ='%s' and month(BREAKDOWN_DATE) = '%s' and\n BREAKDOWN_STK_HOLD_ID ='%d' and STATION_ID_CID_TRIGGER= '%s'" ("condition")) -> (w467:string)
              n112 = Concatenate Strings("Select BREAKDOWN_IN_TIME,BREAKDOWN_OUT_TIME,DATEDIFF(MINUTE,BREAKDOWN_IN_TIME,BREAKDOWN_OUT_TIME)\nfrom STATION_1_LOG_HISTORY\n" ("string"), "Where year(BREAKDOWN_DATE) ='%s' and month(BREAKDOWN_DATE) = '%s' and\n BREAKDOWN_STK_HOLD_ID ='%d' and STATION_ID_CID_TRIGGER= '%s'" ("condition")) -> (w461:string)
              n113 = for {
                tunnel: w468 -> [w491]
                tunnel: w467 -> [w490]
                tunnel: w465 -> [w488]
                tunnel: w464 -> [w487]
                tunnel: [w486] -> w463
                tunnel: w462 -> [w485]
                shift-right: [w483] -> w469
                shift-left: string[][] [] ("Output Array") -> [w489]
                tunnel: w461 -> [w481]
                tunnel: [w480] -> w458
                shift-right: [w476] -> w459
                shift-left: string[][] [] ("Output Array") -> [w477]
                tunnel: [w475] -> w455
                tunnel: w456 -> [w474]
                tunnel: "2" -> [w473]
                n114 = for {
                  tunnel: w490 -> [w513]
                  tunnel: w491 -> [w503]
                  tunnel: w488 -> [w502]
                  tunnel: [w512] -> _ mode=indexing
                  tunnel: w487 -> [w500]
                  tunnel: [w510] -> w486
                  tunnel: w485 -> [w501] mode=indexing
                  shift-right: [w511] -> w484
                  shift-left: w489 -> [w511]
                  tunnel: [w506] -> w482 mode=indexing
                  tunnel: w481 -> [w504]
                  tunnel: [w497] -> w480
                  tunnel: [w496] -> w479 mode=indexing
                  shift-right: [w495] -> w478
                  shift-left: w477 -> [w495]
                  tunnel: [w493] -> w475
                  tunnel: w474 -> [w493]
                  tunnel: w473 -> [w492]
                  n115 = Format Into String(format string=w504, w503, w502, w501, w492) -> (resulting string=w505:string)  [unwired: 2 in, 1 out]
                  n116 = Format Into String(format string=w513, w503, w502, w501, w492) -> (resulting string=w512:string)  [unwired: 2 in, 1 out]
                  n117 = call "Execute query.vi"("String"=w512, "connection reference"=w500) -> ("Table"=w509:string[][], "connection reference 2"=w510:T1)  [unwired: 6 in, 2 out]
                  n118 = call "Execute query.vi"("String"=w505, "connection reference"=w500) -> ("Table"=w499:string[][], "connection reference 2"=w497:T1)  [unwired: 6 in, 2 out]
                  n119 = Index Array(array=w509, index (row)=0 ("disabled index (col)")) -> (element=w507:string[])  [unwired: 1 in]
                  n120 = Index Array(array=w499, index (col)=2 ("disabled index (col)")) -> (element=w498:string[])  [unwired: 1 in]
                  n121 = Index Array(array=w498) -> (element=w496:string)  [unwired: 1 in]
                  n122 = Index Array(array=w507) -> (element=w506:string)  [unwired: 1 in]
                }
                n123 = Build Array (concatenate)(w484, w482) -> (w483:string[][])
                n124 = Build Array (concatenate)(w478, w479) -> (w476:string[][])
              }
            }
            frame "1" {
              n125 = Array Size() -> (size(s)=w528:i32)  [unwired: 1 in]
              n126 = Concatenate Strings("select count(BREAKDOWN_STK_HOLD_ID) from " ("string"), "STATION_1_LOG_HISTORY" ("table"), "\n" ("string"), "Where year(BREAKDOWN_DATE) ='%s' and month(BREAKDOWN_DATE) = '%s' and\n BREAKDOWN_STK_HOLD_ID ='%d' and STATION_ID_CID_TRIGGER= '%s'and\nSHIFT_ID='%s'" ("condition")) -> (w530:string)
              n127 = Concatenate Strings("Select BREAKDOWN_IN_TIME,BREAKDOWN_OUT_TIME,DATEDIFF(MINUTE,BREAKDOWN_IN_TIME,BREAKDOWN_OUT_TIME)\nfrom STATION_1_LOG_HISTORY\n\n" ("string"), "Where year(BREAKDOWN_DATE) ='%s' and month(BREAKDOWN_DATE) = '%s' and\n BREAKDOWN_STK_HOLD_ID ='%d' and STATION_ID_CID_TRIGGER= '%s'and\nSHIFT_ID='%s'" ("condition")) -> (w521:string)
              n128 = for {
                tunnel: w531 -> [w555]
                tunnel: w530 -> [w554]
                tunnel: w528 -> [w552]
                tunnel: w527 -> [w551]
                tunnel: [w550] -> w526
                tunnel: w525 -> [w549]
                shift-right: [w547] -> w532
                shift-left: string[][] [] ("Output Array") -> [w553]
                tunnel: w521 -> [w545]
                shift-right: [w541] -> w523
                shift-left: string[][] [] ("Output Array") -> [w543]
                tunnel: [w540] -> w522
                tunnel: "2" -> [w539]
                tunnel: w517 -> [w538]
                tunnel: [w537] -> w515
                tunnel: w514 -> [w536]
                n129 = for {
                  tunnel: w554 -> [w577]
                  tunnel: w555 -> [w565]
                  tunnel: [w576] -> _ mode=indexing
                  tunnel: w552 -> [_]
                  tunnel: w551 -> [w561]
                  tunnel: [w574] -> w550
                  tunnel: w549 -> [w564] mode=indexing
                  shift-right: [w575] -> w548
                  shift-left: w553 -> [w575]
                  tunnel: [w571] -> w546 mode=indexing
                  tunnel: w545 -> [w566]
                  tunnel: [w563] -> w544 mode=indexing
                  shift-right: [w562] -> w542
                  shift-left: w543 -> [w562]
                  tunnel: [w560] -> w540
                  tunnel: w539 -> [w558]
                  tunnel: w538 -> [w557]
                  tunnel: [w556] -> w537
                  tunnel: w536 -> [w556]
                  n130 = Format Into String(format string=w577, w565, w564, w558, w557) -> (resulting string=w576:string)  [unwired: 3 in, 1 out]
                  n131 = Format Into String(format string=w566, w565, w564, w558, w557) -> (resulting string=w569:string)  [unwired: 3 in, 1 out]
                  n132 = call "Execute query.vi"("String"=w576, "connection reference"=w561) -> ("Table"=w570:string[][], "connection reference 2"=w574:T1)  [unwired: 6 in, 2 out]
                  n133 = call "Execute query.vi"("String"=w569, "connection reference"=w561) -> ("Table"=w567:string[][], "connection reference 2"=w560:T1)  [unwired: 6 in, 2 out]
                  n134 = Index Array(array=w570, index (row)=0 ("disabled index (col)")) -> (element=w572:string[])  [unwired: 1 in]
                  n135 = Index Array(array=w567, index (col)=2 ("disabled index (col)")) -> (element=w568:string[])  [unwired: 1 in]
                  n136 = Index Array(array=w568) -> (element=w563:string)  [unwired: 1 in]
                  n137 = Index Array(array=w572) -> (element=w571:string)  [unwired: 1 in]
                }
                n138 = Build Array (concatenate)(w548, w546) -> (w547:string[][])
                n139 = Build Array (concatenate)(w542, w544) -> (w541:string[][])
              }
            }
            frame "2" {
              n140 = Array Size() -> (size(s)=w592:i32)  [unwired: 1 in]
              n141 = Concatenate Strings("select count(BREAKDOWN_STK_HOLD_ID) from " ("string"), "STATION_1_LOG_HISTORY" ("table"), "\n" ("string"), "Where year(BREAKDOWN_DATE) ='%s' and month(BREAKDOWN_DATE) = '%s' and\n BREAKDOWN_STK_HOLD_ID ='%d' and STATION_ID_CID_TRIGGER= '%s'and\nSHIFT_ID='%s'" ("condition")) -> (w594:string)
              n142 = Concatenate Strings("Select BREAKDOWN_IN_TIME,BREAKDOWN_OUT_TIME,DATEDIFF(MINUTE,BREAKDOWN_IN_TIME,BREAKDOWN_OUT_TIME)\nfrom STATION_1_LOG_HISTORY\n\n" ("string"), "Where year(BREAKDOWN_DATE) ='%s' and month(BREAKDOWN_DATE) = '%s' and\n BREAKDOWN_STK_HOLD_ID ='%d' and STATION_ID_CID_TRIGGER= '%s'and\nSHIFT_ID='%s'" ("condition")) -> (w585:string)
              n143 = for {
                tunnel: w595 -> [w619]
                tunnel: w594 -> [w618]
                tunnel: w592 -> [w616]
                tunnel: w591 -> [w615]
                tunnel: [w614] -> w590
                tunnel: w589 -> [w613]
                shift-right: [w611] -> w596
                shift-left: string[][] [] ("Output Array") -> [w617]
                tunnel: w585 -> [w609]
                shift-right: [w605] -> w587
                shift-left: string[][] [] ("Output Array") -> [w607]
                tunnel: [w604] -> w586
                tunnel: "2" -> [w603]
                tunnel: w581 -> [w602]
                tunnel: [w601] -> w579
                tunnel: w578 -> [w600]
                n144 = for {
                  tunnel: w618 -> [w641]
                  tunnel: w619 -> [w629]
                  tunnel: [w640] -> _ mode=indexing
                  tunnel: w616 -> [_]
                  tunnel: w615 -> [w625]
                  tunnel: [w638] -> w614
                  tunnel: w613 -> [w628] mode=indexing
                  shift-right: [w639] -> w612
                  shift-left: w617 -> [w639]
                  tunnel: [w635] -> w610 mode=indexing
                  tunnel: w609 -> [w630]
                  tunnel: [w627] -> w608 mode=indexing
                  shift-right: [w626] -> w606
                  shift-left: w607 -> [w626]
                  tunnel: [w624] -> w604
                  tunnel: w603 -> [w622]
                  tunnel: w602 -> [w621]
                  tunnel: [w620] -> w601
                  tunnel: w600 -> [w620]
                  n145 = Format Into String(format string=w641, w629, w628, w622, w621) -> (resulting string=w640:string)  [unwired: 3 in, 1 out]
                  n146 = Format Into String(format string=w630, w629, w628, w622, w621) -> (resulting string=w633:string)  [unwired: 3 in, 1 out]
                  n147 = call "Execute query.vi"("String"=w640, "connection reference"=w625) -> ("Table"=w634:string[][], "connection reference 2"=w638:T1)  [unwired: 6 in, 2 out]
                  n148 = call "Execute query.vi"("String"=w633, "connection reference"=w625) -> ("Table"=w631:string[][], "connection reference 2"=w624:T1)  [unwired: 6 in, 2 out]
                  n149 = Index Array(array=w634, index (row)=0 ("disabled index (col)")) -> (element=w636:string[])  [unwired: 1 in]
                  n150 = Index Array(array=w631, index (col)=2 ("disabled index (col)")) -> (element=w632:string[])  [unwired: 1 in]
                  n151 = Index Array(array=w632) -> (element=w627:string)  [unwired: 1 in]
                  n152 = Index Array(array=w636) -> (element=w635:string)  [unwired: 1 in]
                }
                n153 = Build Array (concatenate)(w612, w610) -> (w611:string[][])
                n154 = Build Array (concatenate)(w606, w608) -> (w605:string[][])
              }
            }
            frame "3" {
              n155 = Array Size() -> (size(s)=w656:i32)  [unwired: 1 in]
              n156 = Concatenate Strings("select count(BREAKDOWN_STK_HOLD_ID) from " ("string"), "STATION_1_LOG_HISTORY" ("table"), "\n" ("string"), "Where year(BREAKDOWN_DATE) ='%s' and month(BREAKDOWN_DATE) = '%s' and\n BREAKDOWN_STK_HOLD_ID ='%d' and STATION_ID_CID_TRIGGER= '%s'and\nSHIFT_ID='%s'" ("condition")) -> (w658:string)
              n157 = Concatenate Strings("Select BREAKDOWN_IN_TIME,BREAKDOWN_OUT_TIME,DATEDIFF(MINUTE,BREAKDOWN_IN_TIME,BREAKDOWN_OUT_TIME)\nfrom STATION_1_LOG_HISTORY\n\n" ("string"), "Where year(BREAKDOWN_DATE) ='%s' and month(BREAKDOWN_DATE) = '%s' and\n BREAKDOWN_STK_HOLD_ID ='%d' and STATION_ID_CID_TRIGGER= '%s'and\nSHIFT_ID='%s'" ("condition")) -> (w649:string)
              n158 = for {
                tunnel: w659 -> [w683]
                tunnel: w658 -> [w682]
                tunnel: w656 -> [w680]
                tunnel: w655 -> [w679]
                tunnel: [w678] -> w654
                tunnel: w653 -> [w677]
                shift-right: [w675] -> w660
                shift-left: string[][] [] ("Output Array") -> [w681]
                tunnel: w649 -> [w673]
                shift-right: [w669] -> w651
                shift-left: string[][] [] ("Output Array") -> [w671]
                tunnel: [w668] -> w650
                tunnel: "2" -> [w667]
                tunnel: w645 -> [w666]
                tunnel: [w665] -> w643
                tunnel: w642 -> [w664]
                n159 = for {
                  tunnel: w682 -> [w705]
                  tunnel: w683 -> [w693]
                  tunnel: [w704] -> _ mode=indexing
                  tunnel: w680 -> [_]
                  tunnel: w679 -> [w689]
                  tunnel: [w702] -> w678
                  tunnel: w677 -> [w692] mode=indexing
                  shift-right: [w703] -> w676
                  shift-left: w681 -> [w703]
                  tunnel: [w699] -> w674 mode=indexing
                  tunnel: w673 -> [w694]
                  tunnel: [w691] -> w672 mode=indexing
                  shift-right: [w690] -> w670
                  shift-left: w671 -> [w690]
                  tunnel: [w688] -> w668
                  tunnel: w667 -> [w686]
                  tunnel: w666 -> [w685]
                  tunnel: [w684] -> w665
                  tunnel: w664 -> [w684]
                  n160 = Format Into String(format string=w705, w693, w692, w686, w685) -> (resulting string=w704:string)  [unwired: 3 in, 1 out]
                  n161 = Format Into String(format string=w694, w693, w692, w686, w685) -> (resulting string=w697:string)  [unwired: 3 in, 1 out]
                  n162 = call "Execute query.vi"("String"=w704, "connection reference"=w689) -> ("Table"=w698:string[][], "connection reference 2"=w702:T1)  [unwired: 6 in, 2 out]
                  n163 = call "Execute query.vi"("String"=w697, "connection reference"=w689) -> ("Table"=w695:string[][], "connection reference 2"=w688:T1)  [unwired: 6 in, 2 out]
                  n164 = Index Array(array=w698, index (row)=0 ("disabled index (col)")) -> (element=w700:string[])  [unwired: 1 in]
                  n165 = Index Array(array=w695, index (col)=2 ("disabled index (col)")) -> (element=w696:string[])  [unwired: 1 in]
                  n166 = Index Array(array=w696) -> (element=w691:string)  [unwired: 1 in]
                  n167 = Index Array(array=w700) -> (element=w699:string)  [unwired: 1 in]
                }
                n168 = Build Array (concatenate)(w676, w674) -> (w675:string[][])
                n169 = Build Array (concatenate)(w670, w672) -> (w669:string[][])
              }
            }
          }
        }
        frame Enabled {
        }
      }
    }
    frame "ST 3" {
      n170 = disable-structure shown="Disabled" {
        disable-tunnel: w717 -> [w729 _]
        disable-tunnel: w716 -> [w728 _]
        disable-tunnel: w715 -> [w727 _]
        disable-tunnel: w714 -> [w726 _]
        disable-tunnel: [w725 _] -> w713
        disable-tunnel: w712 -> [w724 _]
        disable-tunnel: [w723 _] -> w711
        disable-tunnel: w710 -> [w722 _]
        disable-tunnel: [w721 _] -> w709
        disable-tunnel: [w720 _] -> w708
        disable-tunnel: w707 -> [w719 _]
        disable-tunnel: [w718 _] -> w706
        frame Disabled {
          n171 = case shown="\"False\", Default" w729 {
            selector: w729 -> [_ _ w797 w861 w925]
            tunnel: w728 -> [_ _ _ _ _]
            tunnel: w727 -> [_ w748 w811 w875 w939]
            tunnel: w726 -> [_ w745 _ _ _]
            tunnel: [_ w749 w812 w876 w940] -> w725
            tunnel: w724 -> [w731 w744 w807 w871 w935]
            tunnel: [w731 w743 w806 w870 w934] -> w723
            tunnel: w722 -> [_ w742 w805 w869 w933]
            tunnel: [_ w739 w803 w867 w931] -> w721
            tunnel: [_ w738 w802 w866 w930] -> w720
            tunnel: w719 -> [w730 w736 w794 w858 w922]
            tunnel: [w730 w735 w795 w859 w923] -> w718
            frame "False", Default {
            }
            frame "ALL" {
              n172 = Concatenate Strings("select count(BREAKDOWN_STK_HOLD_ID) from " ("string"), "STATION_1_LOG_HISTORY" ("table"), "\n" ("string"), "Where year(BREAKDOWN_DATE) ='%s' and month(BREAKDOWN_DATE) = '%s' and\n BREAKDOWN_STK_HOLD_ID ='%d' and STATION_ID_CID_TRIGGER= '%s'" ("condition")) -> (w747:string)
              n173 = Concatenate Strings("Select BREAKDOWN_IN_TIME,BREAKDOWN_OUT_TIME,DATEDIFF(MINUTE,BREAKDOWN_IN_TIME,BREAKDOWN_OUT_TIME)\nfrom STATION_1_LOG_HISTORY\n" ("string"), "Where year(BREAKDOWN_DATE) ='%s' and month(BREAKDOWN_DATE) = '%s' and\n BREAKDOWN_STK_HOLD_ID ='%d' and STATION_ID_CID_TRIGGER= '%s'" ("condition")) -> (w741:string)
              n174 = for {
                tunnel: w748 -> [w771]
                tunnel: w747 -> [w770]
                tunnel: w745 -> [w768]
                tunnel: w744 -> [w767]
                tunnel: [w766] -> w743
                tunnel: w742 -> [w765]
                shift-right: [w763] -> w749
                shift-left: string[][] [] ("Output Array") -> [w769]
                tunnel: w741 -> [w761]
                tunnel: [w760] -> w738
                shift-right: [w756] -> w739
                shift-left: string[][] [] ("Output Array") -> [w757]
                tunnel: [w755] -> w735
                tunnel: w736 -> [w754]
                tunnel: "3" -> [w753]
                n175 = for {
                  tunnel: w770 -> [w793]
                  tunnel: w771 -> [w783]
                  tunnel: w768 -> [w782]
                  tunnel: [w792] -> _ mode=indexing
                  tunnel: w767 -> [w780]
                  tunnel: [w790] -> w766
                  tunnel: w765 -> [w781] mode=indexing
                  shift-right: [w791] -> w764
                  shift-left: w769 -> [w791]
                  tunnel: [w786] -> w762 mode=indexing
                  tunnel: w761 -> [w784]
                  tunnel: [w777] -> w760
                  tunnel: [w776] -> w759 mode=indexing
                  shift-right: [w775] -> w758
                  shift-left: w757 -> [w775]
                  tunnel: [w773] -> w755
                  tunnel: w754 -> [w773]
                  tunnel: w753 -> [w772]
                  n176 = Format Into String(format string=w784, w783, w782, w781, w772) -> (resulting string=w785:string)  [unwired: 2 in, 1 out]
                  n177 = Format Into String(format string=w793, w783, w782, w781, w772) -> (resulting string=w792:string)  [unwired: 2 in, 1 out]
                  n178 = call "Execute query.vi"("String"=w792, "connection reference"=w780) -> ("Table"=w789:string[][], "connection reference 2"=w790:T1)  [unwired: 6 in, 2 out]
                  n179 = call "Execute query.vi"("String"=w785, "connection reference"=w780) -> ("Table"=w779:string[][], "connection reference 2"=w777:T1)  [unwired: 6 in, 2 out]
                  n180 = Index Array(array=w789, index (row)=0 ("disabled index (col)")) -> (element=w787:string[])  [unwired: 1 in]
                  n181 = Index Array(array=w779, index (col)=2 ("disabled index (col)")) -> (element=w778:string[])  [unwired: 1 in]
                  n182 = Index Array(array=w778) -> (element=w776:string)  [unwired: 1 in]
                  n183 = Index Array(array=w787) -> (element=w786:string)  [unwired: 1 in]
                }
                n184 = Build Array (concatenate)(w764, w762) -> (w763:string[][])
                n185 = Build Array (concatenate)(w758, w759) -> (w756:string[][])
              }
            }
            frame "1" {
              n186 = Array Size() -> (size(s)=w808:i32)  [unwired: 1 in]
              n187 = Concatenate Strings("select count(BREAKDOWN_STK_HOLD_ID) from " ("string"), "STATION_1_LOG_HISTORY" ("table"), "\n" ("string"), "Where year(BREAKDOWN_DATE) ='%s' and month(BREAKDOWN_DATE) = '%s' and\n BREAKDOWN_STK_HOLD_ID ='%d' and STATION_ID_CID_TRIGGER= '%s'and\nSHIFT_ID='%s'" ("condition")) -> (w810:string)
              n188 = Concatenate Strings("Select BREAKDOWN_IN_TIME,BREAKDOWN_OUT_TIME,DATEDIFF(MINUTE,BREAKDOWN_IN_TIME,BREAKDOWN_OUT_TIME)\nfrom STATION_1_LOG_HISTORY\n\n" ("string"), "Where year(BREAKDOWN_DATE) ='%s' and month(BREAKDOWN_DATE) = '%s' and\n BREAKDOWN_STK_HOLD_ID ='%d' and STATION_ID_CID_TRIGGER= '%s'and\nSHIFT_ID='%s'" ("condition")) -> (w801:string)
              n189 = for {
                tunnel: w811 -> [w835]
                tunnel: w810 -> [w834]
                tunnel: w808 -> [w832]
                tunnel: w807 -> [w831]
                tunnel: [w830] -> w806
                tunnel: w805 -> [w829]
                shift-right: [w827] -> w812
                shift-left: string[][] [] ("Output Array") -> [w833]
                tunnel: w801 -> [w825]
                shift-right: [w821] -> w803
                shift-left: string[][] [] ("Output Array") -> [w823]
                tunnel: [w820] -> w802
                tunnel: "3" -> [w819]
                tunnel: w797 -> [w818]
                tunnel: [w817] -> w795
                tunnel: w794 -> [w816]
                n190 = for {
                  tunnel: w834 -> [w857]
                  tunnel: w835 -> [w845]
                  tunnel: [w856] -> _ mode=indexing
                  tunnel: w832 -> [_]
                  tunnel: w831 -> [w841]
                  tunnel: [w854] -> w830
                  tunnel: w829 -> [w844] mode=indexing
                  shift-right: [w855] -> w828
                  shift-left: w833 -> [w855]
                  tunnel: [w851] -> w826 mode=indexing
                  tunnel: w825 -> [w846]
                  tunnel: [w843] -> w824 mode=indexing
                  shift-right: [w842] -> w822
                  shift-left: w823 -> [w842]
                  tunnel: [w840] -> w820
                  tunnel: w819 -> [w838]
                  tunnel: w818 -> [w837]
                  tunnel: [w836] -> w817
                  tunnel: w816 -> [w836]
                  n191 = Format Into String(format string=w857, w845, w844, w838, w837) -> (resulting string=w856:string)  [unwired: 3 in, 1 out]
                  n192 = Format Into String(format string=w846, w845, w844, w838, w837) -> (resulting string=w849:string)  [unwired: 3 in, 1 out]
                  n193 = call "Execute query.vi"("String"=w856, "connection reference"=w841) -> ("Table"=w850:string[][], "connection reference 2"=w854:T1)  [unwired: 6 in, 2 out]
                  n194 = call "Execute query.vi"("String"=w849, "connection reference"=w841) -> ("Table"=w847:string[][], "connection reference 2"=w840:T1)  [unwired: 6 in, 2 out]
                  n195 = Index Array(array=w850, index (row)=0 ("disabled index (col)")) -> (element=w852:string[])  [unwired: 1 in]
                  n196 = Index Array(array=w847, index (col)=2 ("disabled index (col)")) -> (element=w848:string[])  [unwired: 1 in]
                  n197 = Index Array(array=w848) -> (element=w843:string)  [unwired: 1 in]
                  n198 = Index Array(array=w852) -> (element=w851:string)  [unwired: 1 in]
                }
                n199 = Build Array (concatenate)(w828, w826) -> (w827:string[][])
                n200 = Build Array (concatenate)(w822, w824) -> (w821:string[][])
              }
            }
            frame "2" {
              n201 = Array Size() -> (size(s)=w872:i32)  [unwired: 1 in]
              n202 = Concatenate Strings("select count(BREAKDOWN_STK_HOLD_ID) from " ("string"), "STATION_1_LOG_HISTORY" ("table"), "\n" ("string"), "Where year(BREAKDOWN_DATE) ='%s' and month(BREAKDOWN_DATE) = '%s' and\n BREAKDOWN_STK_HOLD_ID ='%d' and STATION_ID_CID_TRIGGER= '%s'and\nSHIFT_ID='%s'" ("condition")) -> (w874:string)
              n203 = Concatenate Strings("Select BREAKDOWN_IN_TIME,BREAKDOWN_OUT_TIME,DATEDIFF(MINUTE,BREAKDOWN_IN_TIME,BREAKDOWN_OUT_TIME)\nfrom STATION_1_LOG_HISTORY\n\n" ("string"), "Where year(BREAKDOWN_DATE) ='%s' and month(BREAKDOWN_DATE) = '%s' and\n BREAKDOWN_STK_HOLD_ID ='%d' and STATION_ID_CID_TRIGGER= '%s'and\nSHIFT_ID='%s'" ("condition")) -> (w865:string)
              n204 = for {
                tunnel: w875 -> [w899]
                tunnel: w874 -> [w898]
                tunnel: w872 -> [w896]
                tunnel: w871 -> [w895]
                tunnel: [w894] -> w870
                tunnel: w869 -> [w893]
                shift-right: [w891] -> w876
                shift-left: string[][] [] ("Output Array") -> [w897]
                tunnel: w865 -> [w889]
                shift-right: [w885] -> w867
                shift-left: string[][] [] ("Output Array") -> [w887]
                tunnel: [w884] -> w866
                tunnel: "3" -> [w883]
                tunnel: w861 -> [w882]
                tunnel: [w881] -> w859
                tunnel: w858 -> [w880]
                n205 = for {
                  tunnel: w898 -> [w921]
                  tunnel: w899 -> [w909]
                  tunnel: [w920] -> _ mode=indexing
                  tunnel: w896 -> [_]
                  tunnel: w895 -> [w905]
                  tunnel: [w918] -> w894
                  tunnel: w893 -> [w908] mode=indexing
                  shift-right: [w919] -> w892
                  shift-left: w897 -> [w919]
                  tunnel: [w915] -> w890 mode=indexing
                  tunnel: w889 -> [w910]
                  tunnel: [w907] -> w888 mode=indexing
                  shift-right: [w906] -> w886
                  shift-left: w887 -> [w906]
                  tunnel: [w904] -> w884
                  tunnel: w883 -> [w902]
                  tunnel: w882 -> [w901]
                  tunnel: [w900] -> w881
                  tunnel: w880 -> [w900]
                  n206 = Format Into String(format string=w921, w909, w908, w902, w901) -> (resulting string=w920:string)  [unwired: 3 in, 1 out]
                  n207 = Format Into String(format string=w910, w909, w908, w902, w901) -> (resulting string=w913:string)  [unwired: 3 in, 1 out]
                  n208 = call "Execute query.vi"("String"=w920, "connection reference"=w905) -> ("Table"=w914:string[][], "connection reference 2"=w918:T1)  [unwired: 6 in, 2 out]
                  n209 = call "Execute query.vi"("String"=w913, "connection reference"=w905) -> ("Table"=w911:string[][], "connection reference 2"=w904:T1)  [unwired: 6 in, 2 out]
                  n210 = Index Array(array=w914, index (row)=0 ("disabled index (col)")) -> (element=w916:string[])  [unwired: 1 in]
                  n211 = Index Array(array=w911, index (col)=2 ("disabled index (col)")) -> (element=w912:string[])  [unwired: 1 in]
                  n212 = Index Array(array=w912) -> (element=w907:string)  [unwired: 1 in]
                  n213 = Index Array(array=w916) -> (element=w915:string)  [unwired: 1 in]
                }
                n214 = Build Array (concatenate)(w892, w890) -> (w891:string[][])
                n215 = Build Array (concatenate)(w886, w888) -> (w885:string[][])
              }
            }
            frame "3" {
              n216 = Array Size() -> (size(s)=w936:i32)  [unwired: 1 in]
              n217 = Concatenate Strings("select count(BREAKDOWN_STK_HOLD_ID) from " ("string"), "STATION_1_LOG_HISTORY" ("table"), "\n" ("string"), "Where year(BREAKDOWN_DATE) ='%s' and month(BREAKDOWN_DATE) = '%s' and\n BREAKDOWN_STK_HOLD_ID ='%d' and STATION_ID_CID_TRIGGER= '%s'and\nSHIFT_ID='%s'" ("condition")) -> (w938:string)
              n218 = Concatenate Strings("Select BREAKDOWN_IN_TIME,BREAKDOWN_OUT_TIME,DATEDIFF(MINUTE,BREAKDOWN_IN_TIME,BREAKDOWN_OUT_TIME)\nfrom STATION_1_LOG_HISTORY\n\n" ("string"), "Where year(BREAKDOWN_DATE) ='%s' and month(BREAKDOWN_DATE) = '%s' and\n BREAKDOWN_STK_HOLD_ID ='%d' and STATION_ID_CID_TRIGGER= '%s'and\nSHIFT_ID='%s'" ("condition")) -> (w929:string)
              n219 = for {
                tunnel: w939 -> [w963]
                tunnel: w938 -> [w962]
                tunnel: w936 -> [w960]
                tunnel: w935 -> [w959]
                tunnel: [w958] -> w934
                tunnel: w933 -> [w957]
                shift-right: [w955] -> w940
                shift-left: string[][] [] ("Output Array") -> [w961]
                tunnel: w929 -> [w953]
                shift-right: [w949] -> w931
                shift-left: string[][] [] ("Output Array") -> [w951]
                tunnel: [w948] -> w930
                tunnel: "3" -> [w947]
                tunnel: w925 -> [w946]
                tunnel: [w945] -> w923
                tunnel: w922 -> [w944]
                n220 = for {
                  tunnel: w962 -> [w985]
                  tunnel: w963 -> [w973]
                  tunnel: [w984] -> _ mode=indexing
                  tunnel: w960 -> [_]
                  tunnel: w959 -> [w969]
                  tunnel: [w982] -> w958
                  tunnel: w957 -> [w972] mode=indexing
                  shift-right: [w983] -> w956
                  shift-left: w961 -> [w983]
                  tunnel: [w979] -> w954 mode=indexing
                  tunnel: w953 -> [w974]
                  tunnel: [w971] -> w952 mode=indexing
                  shift-right: [w970] -> w950
                  shift-left: w951 -> [w970]
                  tunnel: [w968] -> w948
                  tunnel: w947 -> [w966]
                  tunnel: w946 -> [w965]
                  tunnel: [w964] -> w945
                  tunnel: w944 -> [w964]
                  n221 = Format Into String(format string=w985, w973, w972, w966, w965) -> (resulting string=w984:string)  [unwired: 3 in, 1 out]
                  n222 = Format Into String(format string=w974, w973, w972, w966, w965) -> (resulting string=w977:string)  [unwired: 3 in, 1 out]
                  n223 = call "Execute query.vi"("String"=w984, "connection reference"=w969) -> ("Table"=w978:string[][], "connection reference 2"=w982:T1)  [unwired: 6 in, 2 out]
                  n224 = call "Execute query.vi"("String"=w977, "connection reference"=w969) -> ("Table"=w975:string[][], "connection reference 2"=w968:T1)  [unwired: 6 in, 2 out]
                  n225 = Index Array(array=w978, index (row)=0 ("disabled index (col)")) -> (element=w980:string[])  [unwired: 1 in]
                  n226 = Index Array(array=w975, index (col)=2 ("disabled index (col)")) -> (element=w976:string[])  [unwired: 1 in]
                  n227 = Index Array(array=w976) -> (element=w971:string)  [unwired: 1 in]
                  n228 = Index Array(array=w980) -> (element=w979:string)  [unwired: 1 in]
                }
                n229 = Build Array (concatenate)(w956, w954) -> (w955:string[][])
                n230 = Build Array (concatenate)(w950, w952) -> (w949:string[][])
              }
            }
          }
        }
        frame Enabled {
        }
      }
    }
    frame "ST 4" {
      n231 = disable-structure shown="Disabled" {
        disable-tunnel: w997 -> [w1009 _]
        disable-tunnel: w996 -> [w1008 _]
        disable-tunnel: w995 -> [w1007 _]
        disable-tunnel: w994 -> [w1006 _]
        disable-tunnel: [w1005 _] -> w993
        disable-tunnel: w992 -> [w1004 _]
        disable-tunnel: [w1003 _] -> w991
        disable-tunnel: w990 -> [w1002 _]
        disable-tunnel: [w1001 _] -> w989
        disable-tunnel: [w1000 _] -> w988
        disable-tunnel: w987 -> [w999 _]
        disable-tunnel: [w998 _] -> w986
        frame Disabled {
          n232 = case shown="\"ALL\"" w1009 {
            selector: w1009 -> [_ _ w1077 w1141 w1205]
            tunnel: w1008 -> [_ _ _ _ _]
            tunnel: w1007 -> [_ w1028 w1091 w1155 w1219]
            tunnel: w1006 -> [_ w1025 _ _ _]
            tunnel: [_ w1029 w1092 w1156 w1220] -> w1005
            tunnel: w1004 -> [w1011 w1024 w1087 w1151 w1215]
            tunnel: [w1011 w1023 w1086 w1150 w1214] -> w1003
            tunnel: w1002 -> [_ w1022 w1085 w1149 w1213]
            tunnel: [_ w1019 w1083 w1147 w1211] -> w1001
            tunnel: [_ w1018 w1082 w1146 w1210] -> w1000
            tunnel: w999 -> [w1010 w1016 w1074 w1138 w1202]
            tunnel: [w1010 w1015 w1075 w1139 w1203] -> w998
            frame "False", Default {
            }
            frame "ALL" {
              n233 = Concatenate Strings("select count(BREAKDOWN_STK_HOLD_ID) from " ("string"), "STATION_1_LOG_HISTORY" ("table"), "\n" ("string"), "Where year(BREAKDOWN_DATE) ='%s' and month(BREAKDOWN_DATE) = '%s' and\n BREAKDOWN_STK_HOLD_ID ='%d' and STATION_ID_CID_TRIGGER= '%s'" ("condition")) -> (w1027:string)
              n234 = Concatenate Strings("Select BREAKDOWN_IN_TIME,BREAKDOWN_OUT_TIME,DATEDIFF(MINUTE,BREAKDOWN_IN_TIME,BREAKDOWN_OUT_TIME)\nfrom STATION_1_LOG_HISTORY\n" ("string"), "Where year(BREAKDOWN_DATE) ='%s' and month(BREAKDOWN_DATE) = '%s' and\n BREAKDOWN_STK_HOLD_ID ='%d' and STATION_ID_CID_TRIGGER= '%s'" ("condition")) -> (w1021:string)
              n235 = for {
                tunnel: w1028 -> [w1051]
                tunnel: w1027 -> [w1050]
                tunnel: w1025 -> [w1048]
                tunnel: w1024 -> [w1047]
                tunnel: [w1046] -> w1023
                tunnel: w1022 -> [w1045]
                shift-right: [w1043] -> w1029
                shift-left: string[][] [] ("Output Array") -> [w1049]
                tunnel: w1021 -> [w1041]
                tunnel: [w1040] -> w1018
                shift-right: [w1036] -> w1019
                shift-left: string[][] [] ("Output Array") -> [w1037]
                tunnel: [w1035] -> w1015
                tunnel: w1016 -> [w1034]
                tunnel: "4" -> [w1033]
                n236 = for {
                  tunnel: w1050 -> [w1073]
                  tunnel: w1051 -> [w1063]
                  tunnel: w1048 -> [w1062]
                  tunnel: [w1072] -> _ mode=indexing
                  tunnel: w1047 -> [w1060]
                  tunnel: [w1070] -> w1046
                  tunnel: w1045 -> [w1061] mode=indexing
                  shift-right: [w1071] -> w1044
                  shift-left: w1049 -> [w1071]
                  tunnel: [w1066] -> w1042 mode=indexing
                  tunnel: w1041 -> [w1064]
                  tunnel: [w1057] -> w1040
                  tunnel: [w1056] -> w1039 mode=indexing
                  shift-right: [w1055] -> w1038
                  shift-left: w1037 -> [w1055]
                  tunnel: [w1053] -> w1035
                  tunnel: w1034 -> [w1053]
                  tunnel: w1033 -> [w1052]
                  n237 = Format Into String(format string=w1064, w1063, w1062, w1061, w1052) -> (resulting string=w1065:string)  [unwired: 2 in, 1 out]
                  n238 = Format Into String(format string=w1073, w1063, w1062, w1061, w1052) -> (resulting string=w1072:string)  [unwired: 2 in, 1 out]
                  n239 = call "Execute query.vi"("String"=w1072, "connection reference"=w1060) -> ("Table"=w1069:string[][], "connection reference 2"=w1070:T1)  [unwired: 6 in, 2 out]
                  n240 = call "Execute query.vi"("String"=w1065, "connection reference"=w1060) -> ("Table"=w1059:string[][], "connection reference 2"=w1057:T1)  [unwired: 6 in, 2 out]
                  n241 = Index Array(array=w1069, index (row)=0 ("disabled index (col)")) -> (element=w1067:string[])  [unwired: 1 in]
                  n242 = Index Array(array=w1059, index (col)=2 ("disabled index (col)")) -> (element=w1058:string[])  [unwired: 1 in]
                  n243 = Index Array(array=w1058) -> (element=w1056:string)  [unwired: 1 in]
                  n244 = Index Array(array=w1067) -> (element=w1066:string)  [unwired: 1 in]
                }
                n245 = Build Array (concatenate)(w1044, w1042) -> (w1043:string[][])
                n246 = Build Array (concatenate)(w1038, w1039) -> (w1036:string[][])
              }
            }
            frame "1" {
              n247 = Array Size() -> (size(s)=w1088:i32)  [unwired: 1 in]
              n248 = Concatenate Strings("select count(BREAKDOWN_STK_HOLD_ID) from " ("string"), "STATION_1_LOG_HISTORY" ("table"), "\n" ("string"), "Where year(BREAKDOWN_DATE) ='%s' and month(BREAKDOWN_DATE) = '%s' and\n BREAKDOWN_STK_HOLD_ID ='%d' and STATION_ID_CID_TRIGGER= '%s'and\nSHIFT_ID='%s'" ("condition")) -> (w1090:string)
              n249 = Concatenate Strings("Select BREAKDOWN_IN_TIME,BREAKDOWN_OUT_TIME,DATEDIFF(MINUTE,BREAKDOWN_IN_TIME,BREAKDOWN_OUT_TIME)\nfrom STATION_1_LOG_HISTORY\n\n" ("string"), "Where year(BREAKDOWN_DATE) ='%s' and month(BREAKDOWN_DATE) = '%s' and\n BREAKDOWN_STK_HOLD_ID ='%d' and STATION_ID_CID_TRIGGER= '%s'and\nSHIFT_ID='%s'" ("condition")) -> (w1081:string)
              n250 = for {
                tunnel: w1091 -> [w1115]
                tunnel: w1090 -> [w1114]
                tunnel: w1088 -> [w1112]
                tunnel: w1087 -> [w1111]
                tunnel: [w1110] -> w1086
                tunnel: w1085 -> [w1109]
                shift-right: [w1107] -> w1092
                shift-left: string[][] [] ("Output Array") -> [w1113]
                tunnel: w1081 -> [w1105]
                shift-right: [w1101] -> w1083
                shift-left: string[][] [] ("Output Array") -> [w1103]
                tunnel: [w1100] -> w1082
                tunnel: "4" -> [w1099]
                tunnel: w1077 -> [w1098]
                tunnel: [w1097] -> w1075
                tunnel: w1074 -> [w1096]
                n251 = for {
                  tunnel: w1114 -> [w1137]
                  tunnel: w1115 -> [w1125]
                  tunnel: [w1136] -> _ mode=indexing
                  tunnel: w1112 -> [_]
                  tunnel: w1111 -> [w1121]
                  tunnel: [w1134] -> w1110
                  tunnel: w1109 -> [w1124] mode=indexing
                  shift-right: [w1135] -> w1108
                  shift-left: w1113 -> [w1135]
                  tunnel: [w1131] -> w1106 mode=indexing
                  tunnel: w1105 -> [w1126]
                  tunnel: [w1123] -> w1104 mode=indexing
                  shift-right: [w1122] -> w1102
                  shift-left: w1103 -> [w1122]
                  tunnel: [w1120] -> w1100
                  tunnel: w1099 -> [w1118]
                  tunnel: w1098 -> [w1117]
                  tunnel: [w1116] -> w1097
                  tunnel: w1096 -> [w1116]
                  n252 = Format Into String(format string=w1137, w1125, w1124, w1118, w1117) -> (resulting string=w1136:string)  [unwired: 3 in, 1 out]
                  n253 = Format Into String(format string=w1126, w1125, w1124, w1118, w1117) -> (resulting string=w1129:string)  [unwired: 3 in, 1 out]
                  n254 = call "Execute query.vi"("String"=w1136, "connection reference"=w1121) -> ("Table"=w1130:string[][], "connection reference 2"=w1134:T1)  [unwired: 6 in, 2 out]
                  n255 = call "Execute query.vi"("String"=w1129, "connection reference"=w1121) -> ("Table"=w1127:string[][], "connection reference 2"=w1120:T1)  [unwired: 6 in, 2 out]
                  n256 = Index Array(array=w1130, index (row)=0 ("disabled index (col)")) -> (element=w1132:string[])  [unwired: 1 in]
                  n257 = Index Array(array=w1127, index (col)=2 ("disabled index (col)")) -> (element=w1128:string[])  [unwired: 1 in]
                  n258 = Index Array(array=w1128) -> (element=w1123:string)  [unwired: 1 in]
                  n259 = Index Array(array=w1132) -> (element=w1131:string)  [unwired: 1 in]
                }
                n260 = Build Array (concatenate)(w1108, w1106) -> (w1107:string[][])
                n261 = Build Array (concatenate)(w1102, w1104) -> (w1101:string[][])
              }
            }
            frame "2" {
              n262 = Array Size() -> (size(s)=w1152:i32)  [unwired: 1 in]
              n263 = Concatenate Strings("select count(BREAKDOWN_STK_HOLD_ID) from " ("string"), "STATION_1_LOG_HISTORY" ("table"), "\n" ("string"), "Where year(BREAKDOWN_DATE) ='%s' and month(BREAKDOWN_DATE) = '%s' and\n BREAKDOWN_STK_HOLD_ID ='%d' and STATION_ID_CID_TRIGGER= '%s'and\nSHIFT_ID='%s'" ("condition")) -> (w1154:string)
              n264 = Concatenate Strings("Select BREAKDOWN_IN_TIME,BREAKDOWN_OUT_TIME,DATEDIFF(MINUTE,BREAKDOWN_IN_TIME,BREAKDOWN_OUT_TIME)\nfrom STATION_1_LOG_HISTORY\n\n" ("string"), "Where year(BREAKDOWN_DATE) ='%s' and month(BREAKDOWN_DATE) = '%s' and\n BREAKDOWN_STK_HOLD_ID ='%d' and STATION_ID_CID_TRIGGER= '%s'and\nSHIFT_ID='%s'" ("condition")) -> (w1145:string)
              n265 = for {
                tunnel: w1155 -> [w1179]
                tunnel: w1154 -> [w1178]
                tunnel: w1152 -> [w1176]
                tunnel: w1151 -> [w1175]
                tunnel: [w1174] -> w1150
                tunnel: w1149 -> [w1173]
                shift-right: [w1171] -> w1156
                shift-left: string[][] [] ("Output Array") -> [w1177]
                tunnel: w1145 -> [w1169]
                shift-right: [w1165] -> w1147
                shift-left: string[][] [] ("Output Array") -> [w1167]
                tunnel: [w1164] -> w1146
                tunnel: "4" -> [w1163]
                tunnel: w1141 -> [w1162]
                tunnel: [w1161] -> w1139
                tunnel: w1138 -> [w1160]
                n266 = for {
                  tunnel: w1178 -> [w1201]
                  tunnel: w1179 -> [w1189]
                  tunnel: [w1200] -> _ mode=indexing
                  tunnel: w1176 -> [_]
                  tunnel: w1175 -> [w1185]
                  tunnel: [w1198] -> w1174
                  tunnel: w1173 -> [w1188] mode=indexing
                  shift-right: [w1199] -> w1172
                  shift-left: w1177 -> [w1199]
                  tunnel: [w1195] -> w1170 mode=indexing
                  tunnel: w1169 -> [w1190]
                  tunnel: [w1187] -> w1168 mode=indexing
                  shift-right: [w1186] -> w1166
                  shift-left: w1167 -> [w1186]
                  tunnel: [w1184] -> w1164
                  tunnel: w1163 -> [w1182]
                  tunnel: w1162 -> [w1181]
                  tunnel: [w1180] -> w1161
                  tunnel: w1160 -> [w1180]
                  n267 = Format Into String(format string=w1201, w1189, w1188, w1182, w1181) -> (resulting string=w1200:string)  [unwired: 3 in, 1 out]
                  n268 = Format Into String(format string=w1190, w1189, w1188, w1182, w1181) -> (resulting string=w1193:string)  [unwired: 3 in, 1 out]
                  n269 = call "Execute query.vi"("String"=w1200, "connection reference"=w1185) -> ("Table"=w1194:string[][], "connection reference 2"=w1198:T1)  [unwired: 6 in, 2 out]
                  n270 = call "Execute query.vi"("String"=w1193, "connection reference"=w1185) -> ("Table"=w1191:string[][], "connection reference 2"=w1184:T1)  [unwired: 6 in, 2 out]
                  n271 = Index Array(array=w1194, index (row)=0 ("disabled index (col)")) -> (element=w1196:string[])  [unwired: 1 in]
                  n272 = Index Array(array=w1191, index (col)=2 ("disabled index (col)")) -> (element=w1192:string[])  [unwired: 1 in]
                  n273 = Index Array(array=w1192) -> (element=w1187:string)  [unwired: 1 in]
                  n274 = Index Array(array=w1196) -> (element=w1195:string)  [unwired: 1 in]
                }
                n275 = Build Array (concatenate)(w1172, w1170) -> (w1171:string[][])
                n276 = Build Array (concatenate)(w1166, w1168) -> (w1165:string[][])
              }
            }
            frame "3" {
              n277 = Array Size() -> (size(s)=w1216:i32)  [unwired: 1 in]
              n278 = Concatenate Strings("select count(BREAKDOWN_STK_HOLD_ID) from " ("string"), "STATION_1_LOG_HISTORY" ("table"), "\n" ("string"), "Where year(BREAKDOWN_DATE) ='%s' and month(BREAKDOWN_DATE) = '%s' and\n BREAKDOWN_STK_HOLD_ID ='%d' and STATION_ID_CID_TRIGGER= '%s'and\nSHIFT_ID='%s'" ("condition")) -> (w1218:string)
              n279 = Concatenate Strings("Select BREAKDOWN_IN_TIME,BREAKDOWN_OUT_TIME,DATEDIFF(MINUTE,BREAKDOWN_IN_TIME,BREAKDOWN_OUT_TIME)\nfrom STATION_1_LOG_HISTORY\n\n" ("string"), "Where year(BREAKDOWN_DATE) ='%s' and month(BREAKDOWN_DATE) = '%s' and\n BREAKDOWN_STK_HOLD_ID ='%d' and STATION_ID_CID_TRIGGER= '%s'and\nSHIFT_ID='%s'" ("condition")) -> (w1209:string)
              n280 = for {
                tunnel: w1219 -> [w1243]
                tunnel: w1218 -> [w1242]
                tunnel: w1216 -> [w1240]
                tunnel: w1215 -> [w1239]
                tunnel: [w1238] -> w1214
                tunnel: w1213 -> [w1237]
                shift-right: [w1235] -> w1220
                shift-left: string[][] [] ("Output Array") -> [w1241]
                tunnel: w1209 -> [w1233]
                shift-right: [w1229] -> w1211
                shift-left: string[][] [] ("Output Array") -> [w1231]
                tunnel: [w1228] -> w1210
                tunnel: "4" -> [w1227]
                tunnel: w1205 -> [w1226]
                tunnel: [w1225] -> w1203
                tunnel: w1202 -> [w1224]
                n281 = for {
                  tunnel: w1242 -> [w1265]
                  tunnel: w1243 -> [w1253]
                  tunnel: [w1264] -> _ mode=indexing
                  tunnel: w1240 -> [_]
                  tunnel: w1239 -> [w1249]
                  tunnel: [w1262] -> w1238
                  tunnel: w1237 -> [w1252] mode=indexing
                  shift-right: [w1263] -> w1236
                  shift-left: w1241 -> [w1263]
                  tunnel: [w1259] -> w1234 mode=indexing
                  tunnel: w1233 -> [w1254]
                  tunnel: [w1251] -> w1232 mode=indexing
                  shift-right: [w1250] -> w1230
                  shift-left: w1231 -> [w1250]
                  tunnel: [w1248] -> w1228
                  tunnel: w1227 -> [w1246]
                  tunnel: w1226 -> [w1245]
                  tunnel: [w1244] -> w1225
                  tunnel: w1224 -> [w1244]
                  n282 = Format Into String(format string=w1265, w1253, w1252, w1246, w1245) -> (resulting string=w1264:string)  [unwired: 3 in, 1 out]
                  n283 = Format Into String(format string=w1254, w1253, w1252, w1246, w1245) -> (resulting string=w1257:string)  [unwired: 3 in, 1 out]
                  n284 = call "Execute query.vi"("String"=w1264, "connection reference"=w1249) -> ("Table"=w1258:string[][], "connection reference 2"=w1262:T1)  [unwired: 6 in, 2 out]
                  n285 = call "Execute query.vi"("String"=w1257, "connection reference"=w1249) -> ("Table"=w1255:string[][], "connection reference 2"=w1248:T1)  [unwired: 6 in, 2 out]
                  n286 = Index Array(array=w1258, index (row)=0 ("disabled index (col)")) -> (element=w1260:string[])  [unwired: 1 in]
                  n287 = Index Array(array=w1255, index (col)=2 ("disabled index (col)")) -> (element=w1256:string[])  [unwired: 1 in]
                  n288 = Index Array(array=w1256) -> (element=w1251:string)  [unwired: 1 in]
                  n289 = Index Array(array=w1260) -> (element=w1259:string)  [unwired: 1 in]
                }
                n290 = Build Array (concatenate)(w1236, w1234) -> (w1235:string[][])
                n291 = Build Array (concatenate)(w1230, w1232) -> (w1229:string[][])
              }
            }
          }
        }
        frame Enabled {
        }
      }
    }
    frame "ST 5" {
      n292 = disable-structure shown="Disabled" {
        disable-tunnel: w1277 -> [w1289 _]
        disable-tunnel: w1276 -> [w1288 _]
        disable-tunnel: w1275 -> [w1287 _]
        disable-tunnel: w1274 -> [w1286 _]
        disable-tunnel: [w1285 _] -> w1273
        disable-tunnel: w1272 -> [w1284 _]
        disable-tunnel: [w1283 _] -> w1271
        disable-tunnel: w1270 -> [w1282 _]
        disable-tunnel: [w1281 _] -> w1269
        disable-tunnel: [w1280 _] -> w1268
        disable-tunnel: w1267 -> [w1279 _]
        disable-tunnel: [w1278 _] -> w1266
        frame Disabled {
          n293 = case shown="\"1\"" w1289 {
            selector: w1289 -> [_ _ w1358 w1424 w1488]
            tunnel: w1288 -> [_ _ _ _ _]
            tunnel: w1287 -> [_ w1308 w1372 w1438 w1502]
            tunnel: w1286 -> [_ w1305 w1354 _ _]
            tunnel: [_ w1309 w1373 w1439 w1503] -> w1285
            tunnel: w1284 -> [w1291 w1304 w1368 w1434 w1498]
            tunnel: [w1291 w1303 w1367 w1433 w1497] -> w1283
            tunnel: w1282 -> [_ w1302 w1366 w1432 w1496]
            tunnel: [_ w1299 w1364 w1430 w1494] -> w1281
            tunnel: [_ w1298 w1363 w1429 w1493] -> w1280
            tunnel: w1279 -> [w1290 w1296 w1355 w1421 w1485]
            tunnel: [w1290 w1295 w1356 w1422 w1486] -> w1278
            frame "False", Default {
            }
            frame "ALL" {
              n294 = Concatenate Strings("select count(BREAKDOWN_STK_HOLD_ID) from " ("string"), "STATION_1_LOG_HISTORY" ("table"), "\n" ("string"), "Where year(BREAKDOWN_DATE) ='%s' and month(BREAKDOWN_DATE) = '%s' and\n BREAKDOWN_STK_HOLD_ID ='%d' and STATION_ID_CID_TRIGGER= '%s'" ("condition")) -> (w1307:string)
              n295 = Concatenate Strings("Select BREAKDOWN_IN_TIME,BREAKDOWN_OUT_TIME,DATEDIFF(MINUTE,BREAKDOWN_IN_TIME,BREAKDOWN_OUT_TIME)\nfrom STATION_1_LOG_HISTORY\n" ("string"), "Where year(BREAKDOWN_DATE) ='%s' and month(BREAKDOWN_DATE) = '%s' and\n BREAKDOWN_STK_HOLD_ID ='%d' and STATION_ID_CID_TRIGGER= '%s'" ("condition")) -> (w1301:string)
              n296 = for {
                tunnel: w1308 -> [w1331]
                tunnel: w1307 -> [w1330]
                tunnel: w1305 -> [w1328]
                tunnel: w1304 -> [w1327]
                tunnel: [w1326] -> w1303
                tunnel: w1302 -> [w1325]
                shift-right: [w1323] -> w1309
                shift-left: string[][] [] ("Output Array") -> [w1329]
                tunnel: w1301 -> [w1321]
                tunnel: [w1320] -> w1298
                shift-right: [w1316] -> w1299
                shift-left: string[][] [] ("Output Array") -> [w1317]
                tunnel: [w1315] -> w1295
                tunnel: w1296 -> [w1314]
                tunnel: "5" -> [w1313]
                n297 = for {
                  tunnel: w1330 -> [w1353]
                  tunnel: w1331 -> [w1343]
                  tunnel: w1328 -> [w1342]
                  tunnel: [w1352] -> _ mode=indexing
                  tunnel: w1327 -> [w1340]
                  tunnel: [w1350] -> w1326
                  tunnel: w1325 -> [w1341] mode=indexing
                  shift-right: [w1351] -> w1324
                  shift-left: w1329 -> [w1351]
                  tunnel: [w1346] -> w1322 mode=indexing
                  tunnel: w1321 -> [w1344]
                  tunnel: [w1337] -> w1320
                  tunnel: [w1336] -> w1319 mode=indexing
                  shift-right: [w1335] -> w1318
                  shift-left: w1317 -> [w1335]
                  tunnel: [w1333] -> w1315
                  tunnel: w1314 -> [w1333]
                  tunnel: w1313 -> [w1332]
                  n298 = Format Into String(format string=w1344, w1343, w1342, w1341, w1332) -> (resulting string=w1345:string)  [unwired: 2 in, 1 out]
                  n299 = Format Into String(format string=w1353, w1343, w1342, w1341, w1332) -> (resulting string=w1352:string)  [unwired: 2 in, 1 out]
                  n300 = call "Execute query.vi"("String"=w1352, "connection reference"=w1340) -> ("Table"=w1349:string[][], "connection reference 2"=w1350:T1)  [unwired: 6 in, 2 out]
                  n301 = call "Execute query.vi"("String"=w1345, "connection reference"=w1340) -> ("Table"=w1339:string[][], "connection reference 2"=w1337:T1)  [unwired: 6 in, 2 out]
                  n302 = Index Array(array=w1349, index (row)=0 ("disabled index (col)")) -> (element=w1347:string[])  [unwired: 1 in]
                  n303 = Index Array(array=w1339, index (col)=2 ("disabled index (col)")) -> (element=w1338:string[])  [unwired: 1 in]
                  n304 = Index Array(array=w1338) -> (element=w1336:string)  [unwired: 1 in]
                  n305 = Index Array(array=w1347) -> (element=w1346:string)  [unwired: 1 in]
                }
                n306 = Build Array (concatenate)(w1324, w1322) -> (w1323:string[][])
                n307 = Build Array (concatenate)(w1318, w1319) -> (w1316:string[][])
              }
            }
            frame "1" {
              n308 = Array Size() -> (size(s)=w1369:i32)  [unwired: 1 in]
              n309 = Concatenate Strings("select count(BREAKDOWN_STK_HOLD_ID) from " ("string"), "STATION_1_LOG_HISTORY" ("table"), "\n" ("string"), "Where year(BREAKDOWN_DATE) ='%s' and month(BREAKDOWN_DATE) = '%s' and\n BREAKDOWN_STK_HOLD_ID ='%d' and STATION_ID_CID_TRIGGER= '%s'and\nSHIFT_ID='%s'" ("condition")) -> (w1371:string)
              n310 = Concatenate Strings("Select BREAKDOWN_IN_TIME,BREAKDOWN_OUT_TIME,DATEDIFF(MINUTE,BREAKDOWN_IN_TIME,BREAKDOWN_OUT_TIME)\nfrom STATION_1_LOG_HISTORY\n\n" ("string"), "Where year(BREAKDOWN_DATE) ='%s' and month(BREAKDOWN_DATE) = '%s' and\n BREAKDOWN_STK_HOLD_ID ='%d' and STATION_ID_CID_TRIGGER= '%s'and\nSHIFT_ID='%s'" ("condition")) -> (w1362:string)
              n311 = for {
                tunnel: w1372 -> [w1397]
                tunnel: w1371 -> [w1396]
                tunnel: w1369 -> [w1394]
                tunnel: w1368 -> [w1393]
                tunnel: [w1392] -> w1367
                tunnel: w1366 -> [w1391]
                shift-right: [w1389] -> w1373
                shift-left: string[][] [] ("Output Array") -> [w1395]
                tunnel: w1362 -> [w1387]
                shift-right: [w1383] -> w1364
                shift-left: string[][] [] ("Output Array") -> [w1385]
                tunnel: [w1382] -> w1363
                tunnel: "5" -> [w1381]
                tunnel: w1358 -> [w1380]
                tunnel: [w1379] -> w1356
                tunnel: w1355 -> [w1378]
                tunnel: w1354 -> [w1377]
                n312 = for {
                  tunnel: w1396 -> [w1420]
                  tunnel: w1397 -> [w1408]
                  tunnel: [w1419] -> _ mode=indexing
                  tunnel: w1394 -> [_]
                  tunnel: w1393 -> [w1404]
                  tunnel: [w1417] -> w1392
                  tunnel: w1391 -> [w1407] mode=indexing
                  shift-right: [w1418] -> w1390
                  shift-left: w1395 -> [w1418]
                  tunnel: [w1414] -> w1388 mode=indexing
                  tunnel: w1387 -> [w1409]
                  tunnel: [w1406] -> w1386 mode=indexing
                  shift-right: [w1405] -> w1384
                  shift-left: w1385 -> [w1405]
                  tunnel: [w1403] -> w1382
                  tunnel: w1381 -> [w1401]
                  tunnel: w1380 -> [w1400]
                  tunnel: [w1399] -> w1379
                  tunnel: w1378 -> [w1399]
                  tunnel: w1377 -> [w1398]
                  n313 = Format Into String(format string=w1420, w1408, w1398, w1407, w1401, w1400) -> (resulting string=w1419:string)  [unwired: 2 in, 1 out]
                  n314 = Format Into String(format string=w1409, w1408, w1407, w1401, w1400) -> (resulting string=w1412:string)  [unwired: 3 in, 1 out]
                  n315 = call "Execute query.vi"("String"=w1419, "connection reference"=w1404) -> ("Table"=w1413:string[][], "connection reference 2"=w1417:T1)  [unwired: 6 in, 2 out]
                  n316 = call "Execute query.vi"("String"=w1412, "connection reference"=w1404) -> ("Table"=w1410:string[][], "connection reference 2"=w1403:T1)  [unwired: 6 in, 2 out]
                  n317 = Index Array(array=w1413, index (row)=0 ("disabled index (col)")) -> (element=w1415:string[])  [unwired: 1 in]
                  n318 = Index Array(array=w1410, index (col)=2 ("disabled index (col)")) -> (element=w1411:string[])  [unwired: 1 in]
                  n319 = Index Array(array=w1411) -> (element=w1406:string)  [unwired: 1 in]
                  n320 = Index Array(array=w1415) -> (element=w1414:string)  [unwired: 1 in]
                }
                n321 = Build Array (concatenate)(w1390, w1388) -> (w1389:string[][])
                n322 = Build Array (concatenate)(w1384, w1386) -> (w1383:string[][])
              }
            }
            frame "2" {
              n323 = Array Size() -> (size(s)=w1435:i32)  [unwired: 1 in]
              n324 = Concatenate Strings("select count(BREAKDOWN_STK_HOLD_ID) from " ("string"), "STATION_1_LOG_HISTORY" ("table"), "\n" ("string"), "Where year(BREAKDOWN_DATE) ='%s' and month(BREAKDOWN_DATE) = '%s' and\n BREAKDOWN_STK_HOLD_ID ='%d' and STATION_ID_CID_TRIGGER= '%s'and\nSHIFT_ID='%s'" ("condition")) -> (w1437:string)
              n325 = Concatenate Strings("Select BREAKDOWN_IN_TIME,BREAKDOWN_OUT_TIME,DATEDIFF(MINUTE,BREAKDOWN_IN_TIME,BREAKDOWN_OUT_TIME)\nfrom STATION_1_LOG_HISTORY\n\n" ("string"), "Where year(BREAKDOWN_DATE) ='%s' and month(BREAKDOWN_DATE) = '%s' and\n BREAKDOWN_STK_HOLD_ID ='%d' and STATION_ID_CID_TRIGGER= '%s'and\nSHIFT_ID='%s'" ("condition")) -> (w1428:string)
              n326 = for {
                tunnel: w1438 -> [w1462]
                tunnel: w1437 -> [w1461]
                tunnel: w1435 -> [w1459]
                tunnel: w1434 -> [w1458]
                tunnel: [w1457] -> w1433
                tunnel: w1432 -> [w1456]
                shift-right: [w1454] -> w1439
                shift-left: string[][] [] ("Output Array") -> [w1460]
                tunnel: w1428 -> [w1452]
                shift-right: [w1448] -> w1430
                shift-left: string[][] [] ("Output Array") -> [w1450]
                tunnel: [w1447] -> w1429
                tunnel: "5" -> [w1446]
                tunnel: w1424 -> [w1445]
                tunnel: [w1444] -> w1422
                tunnel: w1421 -> [w1443]
                n327 = for {
                  tunnel: w1461 -> [w1484]
                  tunnel: w1462 -> [w1472]
                  tunnel: [w1483] -> _ mode=indexing
                  tunnel: w1459 -> [_]
                  tunnel: w1458 -> [w1468]
                  tunnel: [w1481] -> w1457
                  tunnel: w1456 -> [w1471] mode=indexing
                  shift-right: [w1482] -> w1455
                  shift-left: w1460 -> [w1482]
                  tunnel: [w1478] -> w1453 mode=indexing
                  tunnel: w1452 -> [w1473]
                  tunnel: [w1470] -> w1451 mode=indexing
                  shift-right: [w1469] -> w1449
                  shift-left: w1450 -> [w1469]
                  tunnel: [w1467] -> w1447
                  tunnel: w1446 -> [w1465]
                  tunnel: w1445 -> [w1464]
                  tunnel: [w1463] -> w1444
                  tunnel: w1443 -> [w1463]
                  n328 = Format Into String(format string=w1484, w1472, w1471, w1465, w1464) -> (resulting string=w1483:string)  [unwired: 3 in, 1 out]
                  n329 = Format Into String(format string=w1473, w1472, w1471, w1465, w1464) -> (resulting string=w1476:string)  [unwired: 3 in, 1 out]
                  n330 = call "Execute query.vi"("String"=w1483, "connection reference"=w1468) -> ("Table"=w1477:string[][], "connection reference 2"=w1481:T1)  [unwired: 6 in, 2 out]
                  n331 = call "Execute query.vi"("String"=w1476, "connection reference"=w1468) -> ("Table"=w1474:string[][], "connection reference 2"=w1467:T1)  [unwired: 6 in, 2 out]
                  n332 = Index Array(array=w1477, index (row)=0 ("disabled index (col)")) -> (element=w1479:string[])  [unwired: 1 in]
                  n333 = Index Array(array=w1474, index (col)=2 ("disabled index (col)")) -> (element=w1475:string[])  [unwired: 1 in]
                  n334 = Index Array(array=w1475) -> (element=w1470:string)  [unwired: 1 in]
                  n335 = Index Array(array=w1479) -> (element=w1478:string)  [unwired: 1 in]
                }
                n336 = Build Array (concatenate)(w1455, w1453) -> (w1454:string[][])
                n337 = Build Array (concatenate)(w1449, w1451) -> (w1448:string[][])
              }
            }
            frame "3" {
              n338 = Array Size() -> (size(s)=w1499:i32)  [unwired: 1 in]
              n339 = Concatenate Strings("select count(BREAKDOWN_STK_HOLD_ID) from " ("string"), "STATION_1_LOG_HISTORY" ("table"), "\n" ("string"), "Where year(BREAKDOWN_DATE) ='%s' and month(BREAKDOWN_DATE) = '%s' and\n BREAKDOWN_STK_HOLD_ID ='%d' and STATION_ID_CID_TRIGGER= '%s'and\nSHIFT_ID='%s'" ("condition")) -> (w1501:string)
              n340 = Concatenate Strings("Select BREAKDOWN_IN_TIME,BREAKDOWN_OUT_TIME,DATEDIFF(MINUTE,BREAKDOWN_IN_TIME,BREAKDOWN_OUT_TIME)\nfrom STATION_1_LOG_HISTORY\n\n" ("string"), "Where year(BREAKDOWN_DATE) ='%s' and month(BREAKDOWN_DATE) = '%s' and\n BREAKDOWN_STK_HOLD_ID ='%d' and STATION_ID_CID_TRIGGER= '%s'and\nSHIFT_ID='%s'" ("condition")) -> (w1492:string)
              n341 = for {
                tunnel: w1502 -> [w1526]
                tunnel: w1501 -> [w1525]
                tunnel: w1499 -> [w1523]
                tunnel: w1498 -> [w1522]
                tunnel: [w1521] -> w1497
                tunnel: w1496 -> [w1520]
                shift-right: [w1518] -> w1503
                shift-left: string[][] [] ("Output Array") -> [w1524]
                tunnel: w1492 -> [w1516]
                shift-right: [w1512] -> w1494
                shift-left: string[][] [] ("Output Array") -> [w1514]
                tunnel: [w1511] -> w1493
                tunnel: "5" -> [w1510]
                tunnel: w1488 -> [w1509]
                tunnel: [w1508] -> w1486
                tunnel: w1485 -> [w1507]
                n342 = for {
                  tunnel: w1525 -> [w1548]
                  tunnel: w1526 -> [w1536]
                  tunnel: [w1547] -> _ mode=indexing
                  tunnel: w1523 -> [_]
                  tunnel: w1522 -> [w1532]
                  tunnel: [w1545] -> w1521
                  tunnel: w1520 -> [w1535] mode=indexing
                  shift-right: [w1546] -> w1519
                  shift-left: w1524 -> [w1546]
                  tunnel: [w1542] -> w1517 mode=indexing
                  tunnel: w1516 -> [w1537]
                  tunnel: [w1534] -> w1515 mode=indexing
                  shift-right: [w1533] -> w1513
                  shift-left: w1514 -> [w1533]
                  tunnel: [w1531] -> w1511
                  tunnel: w1510 -> [w1529]
                  tunnel: w1509 -> [w1528]
                  tunnel: [w1527] -> w1508
                  tunnel: w1507 -> [w1527]
                  n343 = Format Into String(format string=w1548, w1536, w1535, w1529, w1528) -> (resulting string=w1547:string)  [unwired: 3 in, 1 out]
                  n344 = Format Into String(format string=w1537, w1536, w1535, w1529, w1528) -> (resulting string=w1540:string)  [unwired: 3 in, 1 out]
                  n345 = call "Execute query.vi"("String"=w1547, "connection reference"=w1532) -> ("Table"=w1541:string[][], "connection reference 2"=w1545:T1)  [unwired: 6 in, 2 out]
                  n346 = call "Execute query.vi"("String"=w1540, "connection reference"=w1532) -> ("Table"=w1538:string[][], "connection reference 2"=w1531:T1)  [unwired: 6 in, 2 out]
                  n347 = Index Array(array=w1541, index (row)=0 ("disabled index (col)")) -> (element=w1543:string[])  [unwired: 1 in]
                  n348 = Index Array(array=w1538, index (col)=2 ("disabled index (col)")) -> (element=w1539:string[])  [unwired: 1 in]
                  n349 = Index Array(array=w1539) -> (element=w1534:string)  [unwired: 1 in]
                  n350 = Index Array(array=w1543) -> (element=w1542:string)  [unwired: 1 in]
                }
                n351 = Build Array (concatenate)(w1519, w1517) -> (w1518:string[][])
                n352 = Build Array (concatenate)(w1513, w1515) -> (w1512:string[][])
              }
            }
          }
        }
        frame Enabled {
        }
      }
    }
    frame "ST 6" {
      n353 = disable-structure shown="Disabled" {
        disable-tunnel: w1560 -> [w1572 _]
        disable-tunnel: w1559 -> [w1571 _]
        disable-tunnel: w1558 -> [w1570 _]
        disable-tunnel: w1557 -> [w1569 _]
        disable-tunnel: [w1568 _] -> w1556
        disable-tunnel: w1555 -> [w1567 _]
        disable-tunnel: [w1566 _] -> w1554
        disable-tunnel: w1553 -> [w1565 _]
        disable-tunnel: [w1564 _] -> w1552
        disable-tunnel: [w1563 _] -> w1551
        disable-tunnel: w1550 -> [w1562 _]
        disable-tunnel: [w1561 _] -> w1549
        frame Disabled {
          n354 = case shown="\"2\"" w1572 {
            selector: w1572 -> [_ _ w1640 w1705 w1769]
            tunnel: w1571 -> [_ _ _ _ _]
            tunnel: w1570 -> [_ w1591 w1654 w1718 w1783]
            tunnel: w1569 -> [_ w1588 _ w1701 _]
            tunnel: [_ w1592 w1655 w1719 w1784] -> w1568
            tunnel: w1567 -> [w1574 w1587 w1650 w1715 w1779]
            tunnel: [w1574 w1586 w1649 w1714 w1778] -> w1566
            tunnel: w1565 -> [_ w1585 w1648 w1713 w1777]
            tunnel: [_ w1582 w1646 w1711 w1775] -> w1564
            tunnel: [_ w1581 w1645 w1710 w1774] -> w1563
            tunnel: w1562 -> [w1573 w1579 w1637 w1702 w1766]
            tunnel: [w1573 w1578 w1638 w1703 w1767] -> w1561
            frame "False", Default {
            }
            frame "ALL" {
              n355 = Concatenate Strings("select count(BREAKDOWN_STK_HOLD_ID) from " ("string"), "STATION_1_LOG_HISTORY" ("table"), "\n" ("string"), "Where year(BREAKDOWN_DATE) ='%s' and month(BREAKDOWN_DATE) = '%s' and\n BREAKDOWN_STK_HOLD_ID ='%d' and STATION_ID_CID_TRIGGER= '%s'" ("condition")) -> (w1590:string)
              n356 = Concatenate Strings("Select BREAKDOWN_IN_TIME,BREAKDOWN_OUT_TIME,DATEDIFF(MINUTE,BREAKDOWN_IN_TIME,BREAKDOWN_OUT_TIME)\nfrom STATION_1_LOG_HISTORY\n" ("string"), "Where year(BREAKDOWN_DATE) ='%s' and month(BREAKDOWN_DATE) = '%s' and\n BREAKDOWN_STK_HOLD_ID ='%d' and STATION_ID_CID_TRIGGER= '%s'" ("condition")) -> (w1584:string)
              n357 = for {
                tunnel: w1591 -> [w1614]
                tunnel: w1590 -> [w1613]
                tunnel: w1588 -> [w1611]
                tunnel: w1587 -> [w1610]
                tunnel: [w1609] -> w1586
                tunnel: w1585 -> [w1608]
                shift-right: [w1606] -> w1592
                shift-left: string[][] [] ("Output Array") -> [w1612]
                tunnel: w1584 -> [w1604]
                tunnel: [w1603] -> w1581
                shift-right: [w1599] -> w1582
                shift-left: string[][] [] ("Output Array") -> [w1600]
                tunnel: [w1598] -> w1578
                tunnel: w1579 -> [w1597]
                tunnel: "6" -> [w1596]
                n358 = for {
                  tunnel: w1613 -> [w1636]
                  tunnel: w1614 -> [w1626]
                  tunnel: w1611 -> [w1625]
                  tunnel: [w1635] -> _ mode=indexing
                  tunnel: w1610 -> [w1623]
                  tunnel: [w1633] -> w1609
                  tunnel: w1608 -> [w1624] mode=indexing
                  shift-right: [w1634] -> w1607
                  shift-left: w1612 -> [w1634]
                  tunnel: [w1629] -> w1605 mode=indexing
                  tunnel: w1604 -> [w1627]
                  tunnel: [w1620] -> w1603
                  tunnel: [w1619] -> w1602 mode=indexing
                  shift-right: [w1618] -> w1601
                  shift-left: w1600 -> [w1618]
                  tunnel: [w1616] -> w1598
                  tunnel: w1597 -> [w1616]
                  tunnel: w1596 -> [w1615]
                  n359 = Format Into String(format string=w1627, w1626, w1625, w1624, w1615) -> (resulting string=w1628:string)  [unwired: 2 in, 1 out]
                  n360 = Format Into String(format string=w1636, w1626, w1625, w1624, w1615) -> (resulting string=w1635:string)  [unwired: 2 in, 1 out]
                  n361 = call "Execute query.vi"("String"=w1635, "connection reference"=w1623) -> ("Table"=w1632:string[][], "connection reference 2"=w1633:T1)  [unwired: 6 in, 2 out]
                  n362 = call "Execute query.vi"("String"=w1628, "connection reference"=w1623) -> ("Table"=w1622:string[][], "connection reference 2"=w1620:T1)  [unwired: 6 in, 2 out]
                  n363 = Index Array(array=w1632, index (row)=0 ("disabled index (col)")) -> (element=w1630:string[])  [unwired: 1 in]
                  n364 = Index Array(array=w1622, index (col)=2 ("disabled index (col)")) -> (element=w1621:string[])  [unwired: 1 in]
                  n365 = Index Array(array=w1621) -> (element=w1619:string)  [unwired: 1 in]
                  n366 = Index Array(array=w1630) -> (element=w1629:string)  [unwired: 1 in]
                }
                n367 = Build Array (concatenate)(w1607, w1605) -> (w1606:string[][])
                n368 = Build Array (concatenate)(w1601, w1602) -> (w1599:string[][])
              }
            }
            frame "1" {
              n369 = Array Size() -> (size(s)=w1651:i32)  [unwired: 1 in]
              n370 = Concatenate Strings("select count(BREAKDOWN_STK_HOLD_ID) from " ("string"), "STATION_1_LOG_HISTORY" ("table"), "\n" ("string"), "Where year(BREAKDOWN_DATE) ='%s' and month(BREAKDOWN_DATE) = '%s' and\n BREAKDOWN_STK_HOLD_ID ='%d' and STATION_ID_CID_TRIGGER= '%s'and\nSHIFT_ID='%s'" ("condition")) -> (w1653:string)
              n371 = Concatenate Strings("Select BREAKDOWN_IN_TIME,BREAKDOWN_OUT_TIME,DATEDIFF(MINUTE,BREAKDOWN_IN_TIME,BREAKDOWN_OUT_TIME)\nfrom STATION_1_LOG_HISTORY\n\n" ("string"), "Where year(BREAKDOWN_DATE) ='%s' and month(BREAKDOWN_DATE) = '%s' and\n BREAKDOWN_STK_HOLD_ID ='%d' and STATION_ID_CID_TRIGGER= '%s'and\nSHIFT_ID='%s'" ("condition")) -> (w1644:string)
              n372 = for {
                tunnel: w1654 -> [w1678]
                tunnel: w1653 -> [w1677]
                tunnel: w1651 -> [w1675]
                tunnel: w1650 -> [w1674]
                tunnel: [w1673] -> w1649
                tunnel: w1648 -> [w1672]
                shift-right: [w1670] -> w1655
                shift-left: string[][] [] ("Output Array") -> [w1676]
                tunnel: w1644 -> [w1668]
                shift-right: [w1664] -> w1646
                shift-left: string[][] [] ("Output Array") -> [w1666]
                tunnel: [w1663] -> w1645
                tunnel: "6" -> [w1662]
                tunnel: w1640 -> [w1661]
                tunnel: [w1660] -> w1638
                tunnel: w1637 -> [w1659]
                n373 = for {
                  tunnel: w1677 -> [w1700]
                  tunnel: w1678 -> [w1688]
                  tunnel: [w1699] -> _ mode=indexing
                  tunnel: w1675 -> [_]
                  tunnel: w1674 -> [w1684]
                  tunnel: [w1697] -> w1673
                  tunnel: w1672 -> [w1687] mode=indexing
                  shift-right: [w1698] -> w1671
                  shift-left: w1676 -> [w1698]
                  tunnel: [w1694] -> w1669 mode=indexing
                  tunnel: w1668 -> [w1689]
                  tunnel: [w1686] -> w1667 mode=indexing
                  shift-right: [w1685] -> w1665
                  shift-left: w1666 -> [w1685]
                  tunnel: [w1683] -> w1663
                  tunnel: w1662 -> [w1681]
                  tunnel: w1661 -> [w1680]
                  tunnel: [w1679] -> w1660
                  tunnel: w1659 -> [w1679]
                  n374 = Format Into String(format string=w1700, w1688, w1687, w1681, w1680) -> (resulting string=w1699:string)  [unwired: 3 in, 1 out]
                  n375 = Format Into String(format string=w1689, w1688, w1687, w1681, w1680) -> (resulting string=w1692:string)  [unwired: 3 in, 1 out]
                  n376 = call "Execute query.vi"("String"=w1699, "connection reference"=w1684) -> ("Table"=w1693:string[][], "connection reference 2"=w1697:T1)  [unwired: 6 in, 2 out]
                  n377 = call "Execute query.vi"("String"=w1692, "connection reference"=w1684) -> ("Table"=w1690:string[][], "connection reference 2"=w1683:T1)  [unwired: 6 in, 2 out]
                  n378 = Index Array(array=w1693, index (row)=0 ("disabled index (col)")) -> (element=w1695:string[])  [unwired: 1 in]
                  n379 = Index Array(array=w1690, index (col)=2 ("disabled index (col)")) -> (element=w1691:string[])  [unwired: 1 in]
                  n380 = Index Array(array=w1691) -> (element=w1686:string)  [unwired: 1 in]
                  n381 = Index Array(array=w1695) -> (element=w1694:string)  [unwired: 1 in]
                }
                n382 = Build Array (concatenate)(w1671, w1669) -> (w1670:string[][])
                n383 = Build Array (concatenate)(w1665, w1667) -> (w1664:string[][])
              }
            }
            frame "2" {
              n384 = Concatenate Strings("select count(BREAKDOWN_STK_HOLD_ID) from " ("string"), "STATION_1_LOG_HISTORY" ("table"), "\n" ("string"), "Where year(BREAKDOWN_DATE) ='%s' and month(BREAKDOWN_DATE) = '%s' and\n BREAKDOWN_STK_HOLD_ID ='%d' and STATION_ID_CID_TRIGGER= '%s'and\nSHIFT_ID='%s'" ("condition")) -> (w1717:string)
              n385 = Concatenate Strings("Select BREAKDOWN_IN_TIME,BREAKDOWN_OUT_TIME,DATEDIFF(MINUTE,BREAKDOWN_IN_TIME,BREAKDOWN_OUT_TIME)\nfrom STATION_1_LOG_HISTORY\n\n" ("string"), "Where year(BREAKDOWN_DATE) ='%s' and month(BREAKDOWN_DATE) = '%s' and\n BREAKDOWN_STK_HOLD_ID ='%d' and STATION_ID_CID_TRIGGER= '%s'and\nSHIFT_ID='%s'" ("condition")) -> (w1709:string)
              n386 = for {
                tunnel: w1718 -> [w1742]
                tunnel: w1717 -> [w1741]
                tunnel: w1701 -> [w1739]
                tunnel: w1715 -> [w1738]
                tunnel: [w1737] -> w1714
                tunnel: w1713 -> [w1736]
                shift-right: [w1734] -> w1719
                shift-left: string[][] [] ("Output Array") -> [w1740]
                tunnel: w1709 -> [w1732]
                shift-right: [w1728] -> w1711
                shift-left: string[][] [] ("Output Array") -> [w1730]
                tunnel: [w1727] -> w1710
                tunnel: "6" -> [w1726]
                tunnel: w1705 -> [w1725]
                tunnel: [w1724] -> w1703
                tunnel: w1702 -> [w1723]
                n387 = for {
                  tunnel: w1741 -> [w1765]
                  tunnel: w1742 -> [w1753]
                  tunnel: w1739 -> [w1752]
                  tunnel: [w1764] -> _ mode=indexing
                  tunnel: w1738 -> [w1748]
                  tunnel: [w1762] -> w1737
                  tunnel: w1736 -> [w1751] mode=indexing
                  shift-right: [w1763] -> w1735
                  shift-left: w1740 -> [w1763]
                  tunnel: [w1759] -> w1733 mode=indexing
                  tunnel: w1732 -> [w1754]
                  tunnel: [w1750] -> w1731 mode=indexing
                  shift-right: [w1749] -> w1729
                  shift-left: w1730 -> [w1749]
                  tunnel: [w1747] -> w1727
                  tunnel: w1726 -> [w1745]
                  tunnel: w1725 -> [w1744]
                  tunnel: [w1743] -> w1724
                  tunnel: w1723 -> [w1743]
                  n388 = Format Into String(format string=w1765, w1753, w1752, w1751, w1745, w1744) -> (resulting string=w1764:string)  [unwired: 2 in, 1 out]
                  n389 = Format Into String(format string=w1754, w1753, w1752, w1751, w1745, w1744) -> (resulting string=w1757:string)  [unwired: 2 in, 1 out]
                  n390 = call "Execute query.vi"("String"=w1764, "connection reference"=w1748) -> ("Table"=w1758:string[][], "connection reference 2"=w1762:T1)  [unwired: 6 in, 2 out]
                  n391 = call "Execute query.vi"("String"=w1757, "connection reference"=w1748) -> ("Table"=w1755:string[][], "connection reference 2"=w1747:T1)  [unwired: 6 in, 2 out]
                  n392 = Index Array(array=w1758, index (row)=0 ("disabled index (col)")) -> (element=w1760:string[])  [unwired: 1 in]
                  n393 = Index Array(array=w1755, index (col)=2 ("disabled index (col)")) -> (element=w1756:string[])  [unwired: 1 in]
                  n394 = Index Array(array=w1756) -> (element=w1750:string)  [unwired: 1 in]
                  n395 = Index Array(array=w1760) -> (element=w1759:string)  [unwired: 1 in]
                }
                n396 = Build Array (concatenate)(w1735, w1733) -> (w1734:string[][])
                n397 = Build Array (concatenate)(w1729, w1731) -> (w1728:string[][])
              }
            }
            frame "3" {
              n398 = Array Size() -> (size(s)=w1780:i32)  [unwired: 1 in]
              n399 = Concatenate Strings("select count(BREAKDOWN_STK_HOLD_ID) from " ("string"), "STATION_1_LOG_HISTORY" ("table"), "\n" ("string"), "Where year(BREAKDOWN_DATE) ='%s' and month(BREAKDOWN_DATE) = '%s' and\n BREAKDOWN_STK_HOLD_ID ='%d' and STATION_ID_CID_TRIGGER= '%s'and\nSHIFT_ID='%s'" ("condition")) -> (w1782:string)
              n400 = Concatenate Strings("Select BREAKDOWN_IN_TIME,BREAKDOWN_OUT_TIME,DATEDIFF(MINUTE,BREAKDOWN_IN_TIME,BREAKDOWN_OUT_TIME)\nfrom STATION_1_LOG_HISTORY\n\n" ("string"), "Where year(BREAKDOWN_DATE) ='%s' and month(BREAKDOWN_DATE) = '%s' and\n BREAKDOWN_STK_HOLD_ID ='%d' and STATION_ID_CID_TRIGGER= '%s'and\nSHIFT_ID='%s'" ("condition")) -> (w1773:string)
              n401 = for {
                tunnel: w1783 -> [w1807]
                tunnel: w1782 -> [w1806]
                tunnel: w1780 -> [w1804]
                tunnel: w1779 -> [w1803]
                tunnel: [w1802] -> w1778
                tunnel: w1777 -> [w1801]
                shift-right: [w1799] -> w1784
                shift-left: string[][] [] ("Output Array") -> [w1805]
                tunnel: w1773 -> [w1797]
                shift-right: [w1793] -> w1775
                shift-left: string[][] [] ("Output Array") -> [w1795]
                tunnel: [w1792] -> w1774
                tunnel: "6" -> [w1791]
                tunnel: w1769 -> [w1790]
                tunnel: [w1789] -> w1767
                tunnel: w1766 -> [w1788]
                n402 = for {
                  tunnel: w1806 -> [w1829]
                  tunnel: w1807 -> [w1817]
                  tunnel: [w1828] -> _ mode=indexing
                  tunnel: w1804 -> [_]
                  tunnel: w1803 -> [w1813]
                  tunnel: [w1826] -> w1802
                  tunnel: w1801 -> [w1816] mode=indexing
                  shift-right: [w1827] -> w1800
                  shift-left: w1805 -> [w1827]
                  tunnel: [w1823] -> w1798 mode=indexing
                  tunnel: w1797 -> [w1818]
                  tunnel: [w1815] -> w1796 mode=indexing
                  shift-right: [w1814] -> w1794
                  shift-left: w1795 -> [w1814]
                  tunnel: [w1812] -> w1792
                  tunnel: w1791 -> [w1810]
                  tunnel: w1790 -> [w1809]
                  tunnel: [w1808] -> w1789
                  tunnel: w1788 -> [w1808]
                  n403 = Format Into String(format string=w1829, w1817, w1816, w1810, w1809) -> (resulting string=w1828:string)  [unwired: 3 in, 1 out]
                  n404 = Format Into String(format string=w1818, w1817, w1816, w1810, w1809) -> (resulting string=w1821:string)  [unwired: 3 in, 1 out]
                  n405 = call "Execute query.vi"("String"=w1828, "connection reference"=w1813) -> ("Table"=w1822:string[][], "connection reference 2"=w1826:T1)  [unwired: 6 in, 2 out]
                  n406 = call "Execute query.vi"("String"=w1821, "connection reference"=w1813) -> ("Table"=w1819:string[][], "connection reference 2"=w1812:T1)  [unwired: 6 in, 2 out]
                  n407 = Index Array(array=w1822, index (row)=0 ("disabled index (col)")) -> (element=w1824:string[])  [unwired: 1 in]
                  n408 = Index Array(array=w1819, index (col)=2 ("disabled index (col)")) -> (element=w1820:string[])  [unwired: 1 in]
                  n409 = Index Array(array=w1820) -> (element=w1815:string)  [unwired: 1 in]
                  n410 = Index Array(array=w1824) -> (element=w1823:string)  [unwired: 1 in]
                }
                n411 = Build Array (concatenate)(w1800, w1798) -> (w1799:string[][])
                n412 = Build Array (concatenate)(w1794, w1796) -> (w1793:string[][])
              }
            }
          }
        }
        frame Enabled {
        }
      }
    }
  }
  "BD Count" <- w9
  "connection reference 2" <- w7
  "error out" <- w3
  "Duration count" <- w5
